vi "calculation vi_MD.vi"() -> ()   [LabVIEW 2012]
uses:
  Custom Controls/display palette control.ctl
  Custom Controls/scan mode main settings tab.ctl
  Custom Controls/pixel resolution enum.ctl
  Custom Controls/speed mode type def.ctl
  <vilib>/Utility/miscctls.llb/LVMinMaxIncTypeDef.ctl
  <vilib>/Utility/miscctls.llb/LVOutOfRangeActionTypeDef.ctl
  Custom Controls/experiment type.ctl
  Custom Controls/advanced settings inner tab CTL.ctl
  Custom Controls/MAIN Image panel tab Control type def.ctl
  Custom Controls/Histogram tab.ctl
  GFG/GFGnumericGet.vi
  GFG/GFGfpRefGet.vi
  GFG/GFGbooleanGet.vi
  GFG/GFGDisplayRefsGet.vi
  GFG/GFGImageRefsGet.vi
  GFG/GFG library.lvlib
panel:
  in  "String":string
  out "ready for flystart?":bool
  out "error out 2":errorcluster
  out "error out":errorcluster
  out "Source VI":string
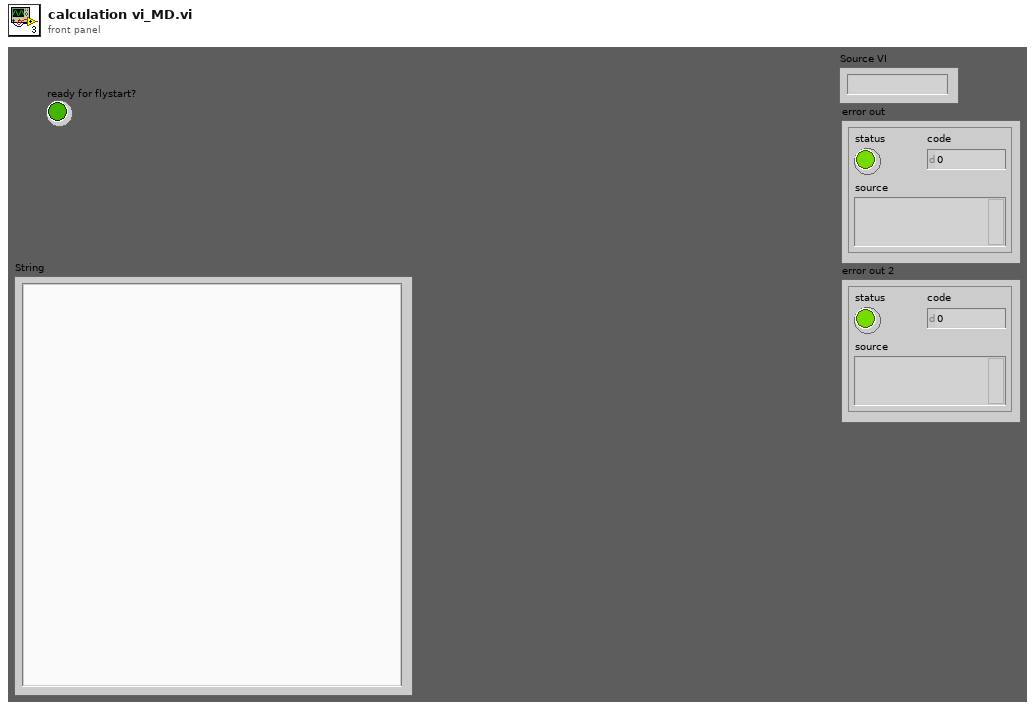
[diagram p1: front panel]
types:
  T1 = typedef "display palette control.ctl" = enum16{"standard", "high clipping red", "low clipping blue", "high and low clipping"}
  T2 = typedef "scan mode main settings tab.ctl" = enum32{"2D frame", "2D line scan", "general settings", "Z Stack", "piezo"}
  T3 = typedef "pixel resolution enum.ctl" = enum16{"   128 x 128", "   256 x 128", "   256 x 256", "   512 x  64", "   512 x 128", "   512 x 256", "   512 x 512", "  1024 x 512", "  1024 x 1024", "   arbitrary"}
  T4 = enum8{"Enabled", "Disabled", "Disabled and Grayed Out"}
  T5 = typedef "LVOutOfRangeActionTypeDef.ctl" = cluster{"Out of Range Action Minimum":u8, "Out of Range Action Maximum":u8, "Out of Range Action Increment":u8}
  T6 = typedef "LVMinMaxIncTypeDef.ctl" = cluster{"Minimum":dbl, "Maximum":dbl, "Increment":dbl}
  T7 = typedef "experiment type.ctl" = string
  T8 = enum32{"Page Enabled", "Page Disabled", "Page Disabled & Grayed"}
  T9 = typedef "advanced settings inner tab CTL.ctl" = enum32{"arb. frames", "AO", "AI", "channels", "trigger", "Zstack data"}
  T10 = typedef "MAIN Image panel tab Control type def.ctl" = enum32{"Channel 1", "Channel 2", "Channel 3", "Channel 4", "all channels", "RGB overlay", "ROI", "arbitrary line scan"}
  T11 = typedef "Histogram tab.ctl" = enum32{"hist Ch 1", "hist Ch 4", "hist Ch 3", "hist Ch 2"}
  T12 = cluster{"WaveformChartRef":refnum<vi>, "DigitalRef":refnum<vi>, "ArrayRef":refnum<vi>, "TabControlRef":refnum<vi>, "EnumRef":refnum<vi>, "RingRef":refnum<vi>, "BooleanRef":refnum<vi>, "KnobRef":refnum<vi>, "SlideRef":refnum<vi>, "PathRef":refnum<vi>, "StringRef":refnum<vi>, "ComboBox":refnum<vi>, "WaveformGraphRef":refnum<vi>}
  T13 = cluster{"Channel 1 small":refnum<vi>, "Channel 2 small":refnum<vi>, "Channel 3 small":refnum<vi>, "Channel 4 small":refnum<vi>, "Channel 1 large":refnum<vi>, "Channel 2 large":refnum<vi>, "Channel 3 large":refnum<vi>, "Channel 4 large":refnum<vi>, "RGB overlay":refnum<vi>, "ROI Image display":refnum<vi>, "arb line scan display":refnum<vi>, "Channel 5 large":refnum<vi>}
  T14 = typedef "IMAQ Image.ctl" = refnum<image>
  T15 = cluster{"Channel 1 small":T14, "Channel 2 small":T14, "Channel 3 small":T14, "Channel 4 small":T14, "Channel 1 large":T14, "Channel 2 large":T14, "Channel 3 large":T14, "Channel 4 large":T14, "RGB overlay":T14, "ROI Image display":T14, "arb line scan display":T14, "Channel 5 large":T14}
  T16 = typedef "speed mode type def.ctl" = u16
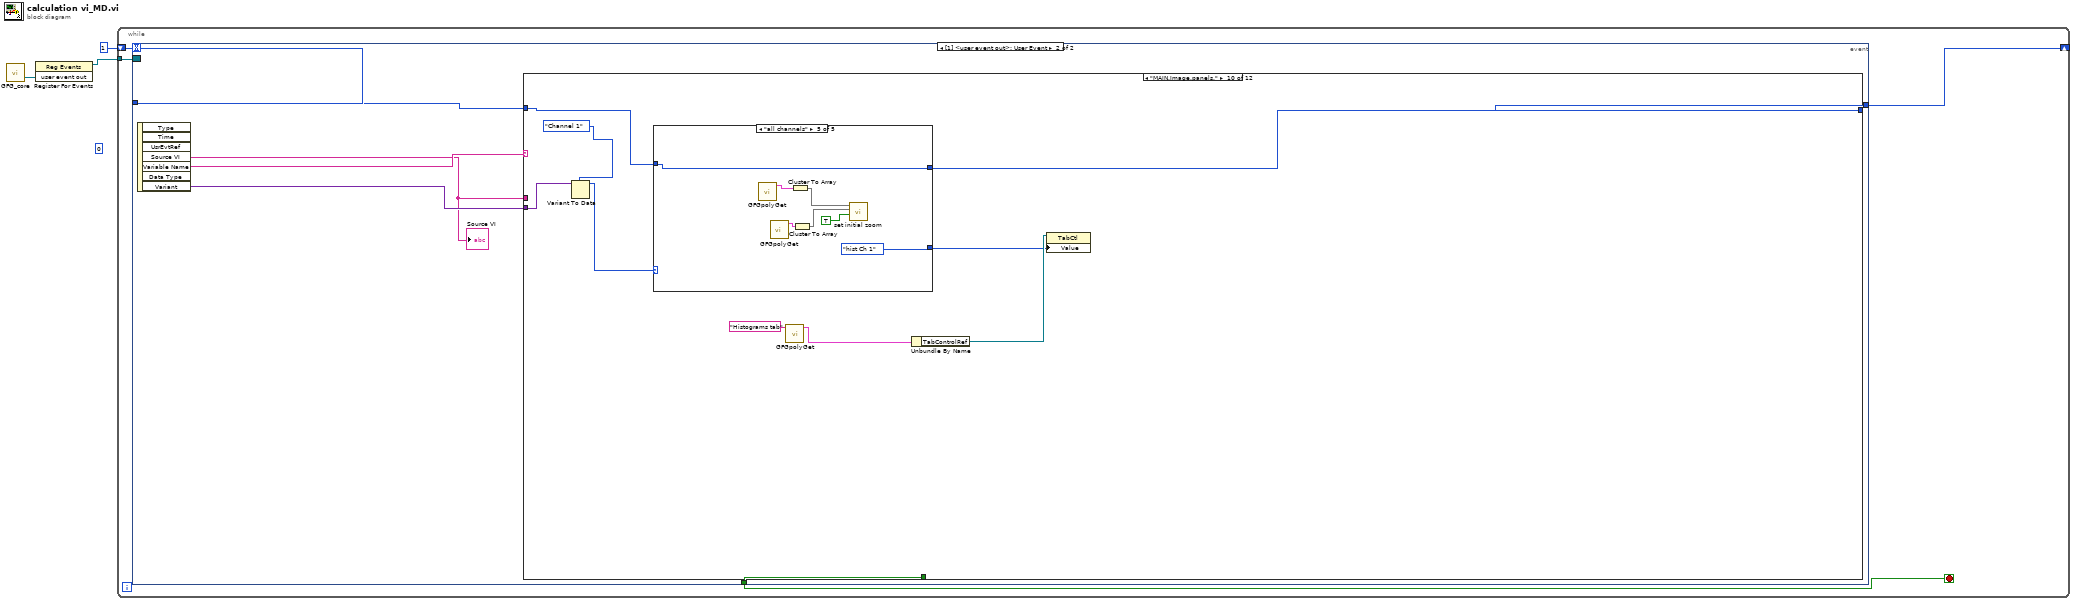
[diagram p0: block diagram]
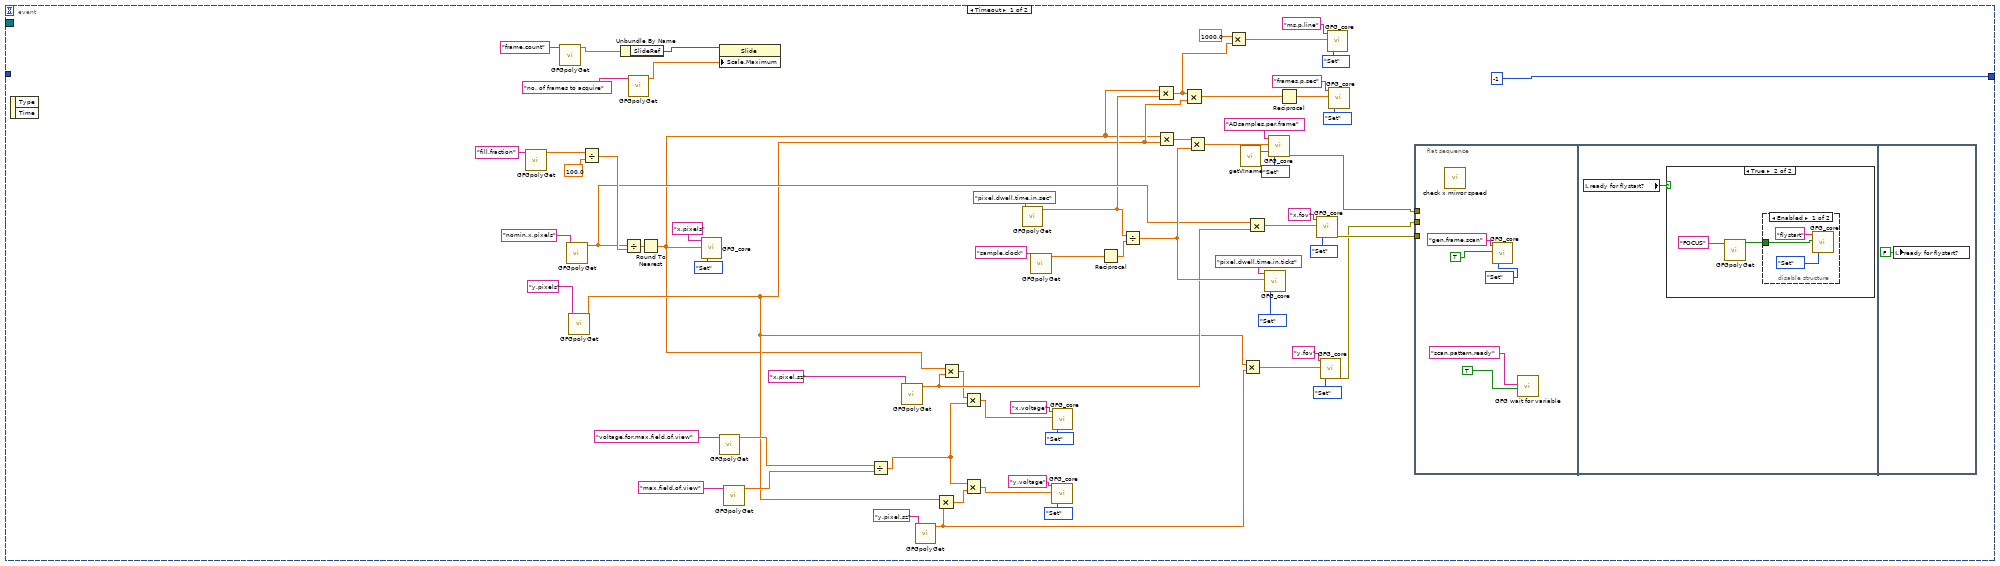
[diagram p2: hidden frame]
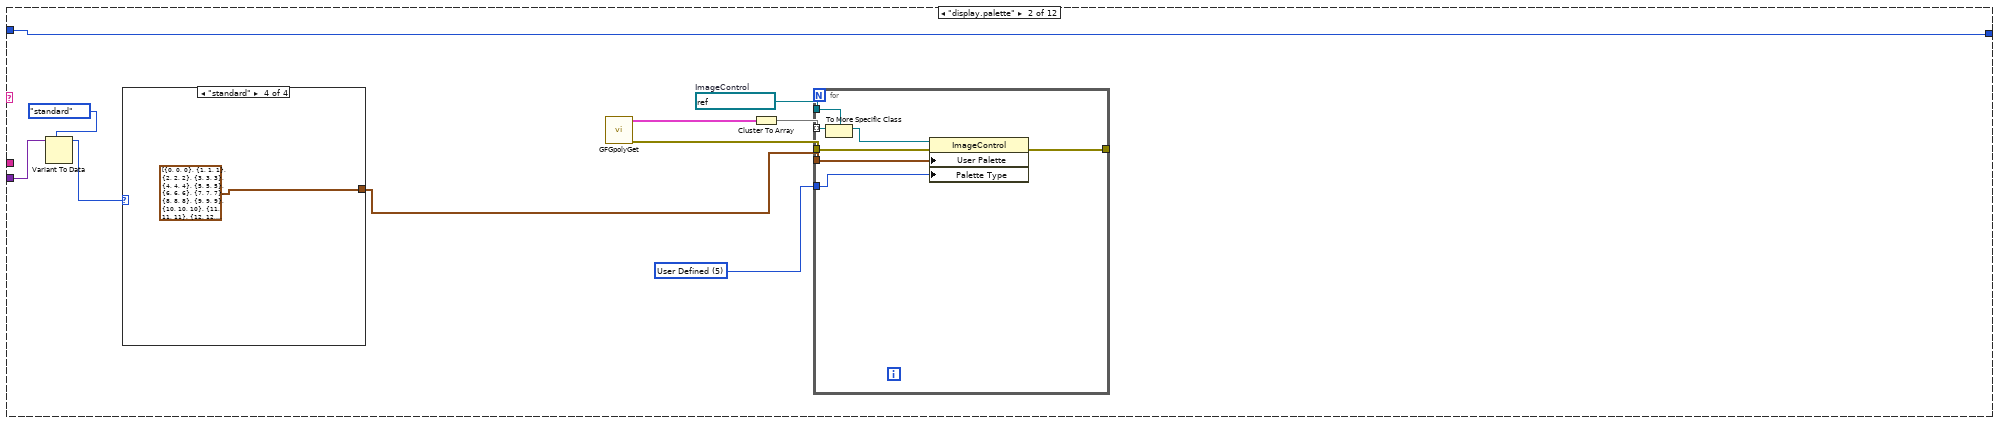
[diagram p6: hidden frame]
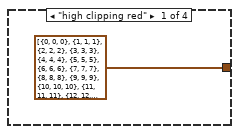
[diagram p7: hidden frame]
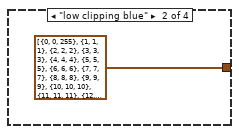
[diagram p8: hidden frame]
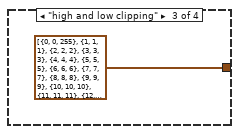
[diagram p9: hidden frame]
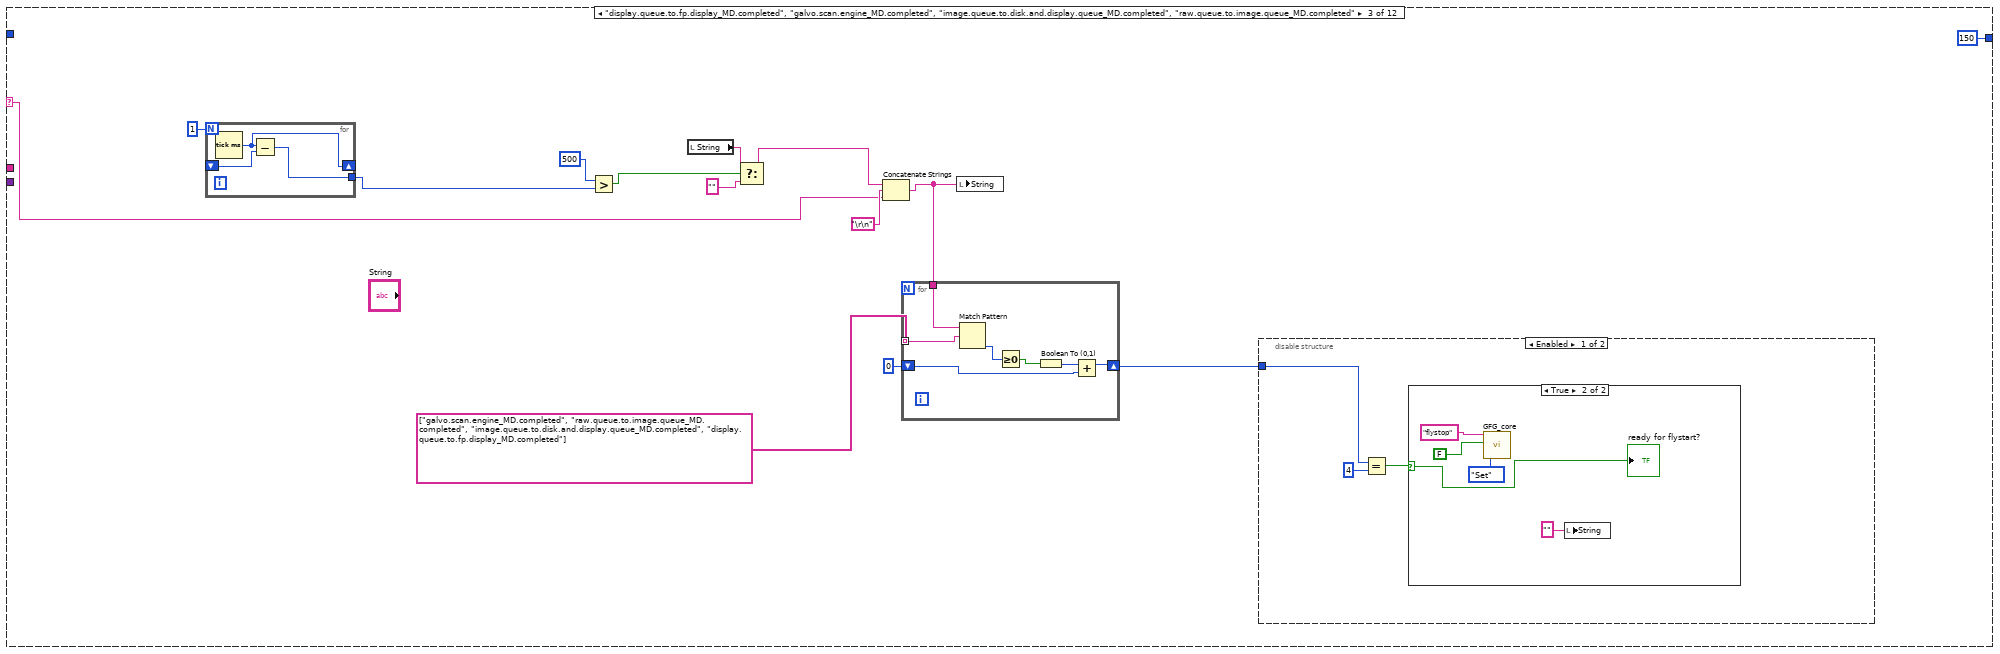
[diagram p10: hidden frame]
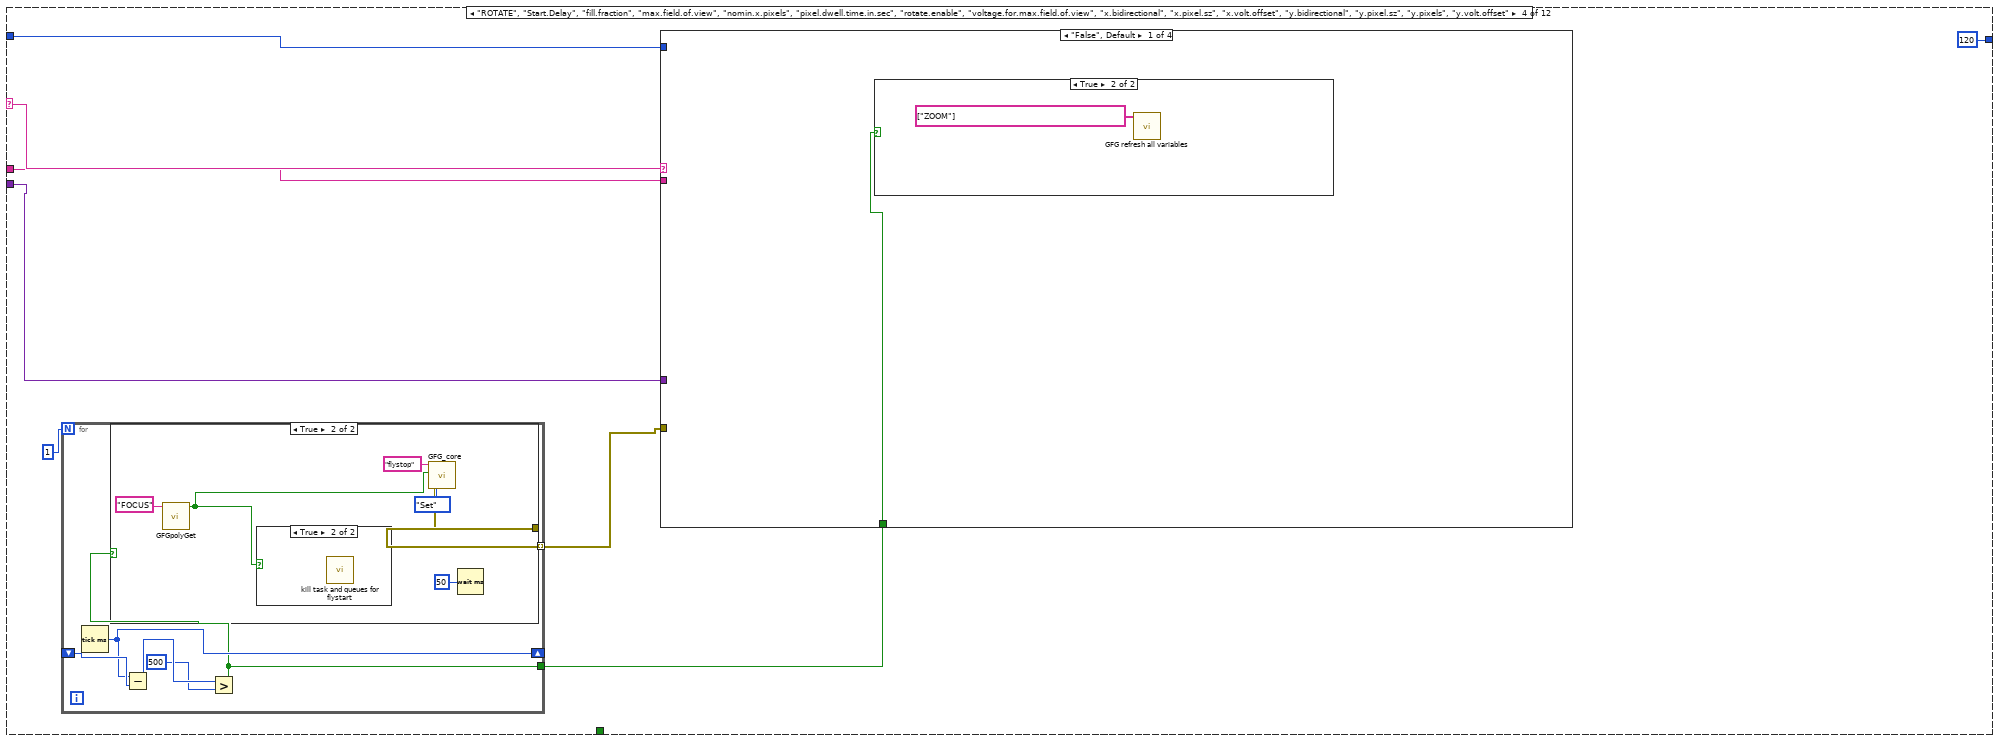
[diagram p13: hidden frame]
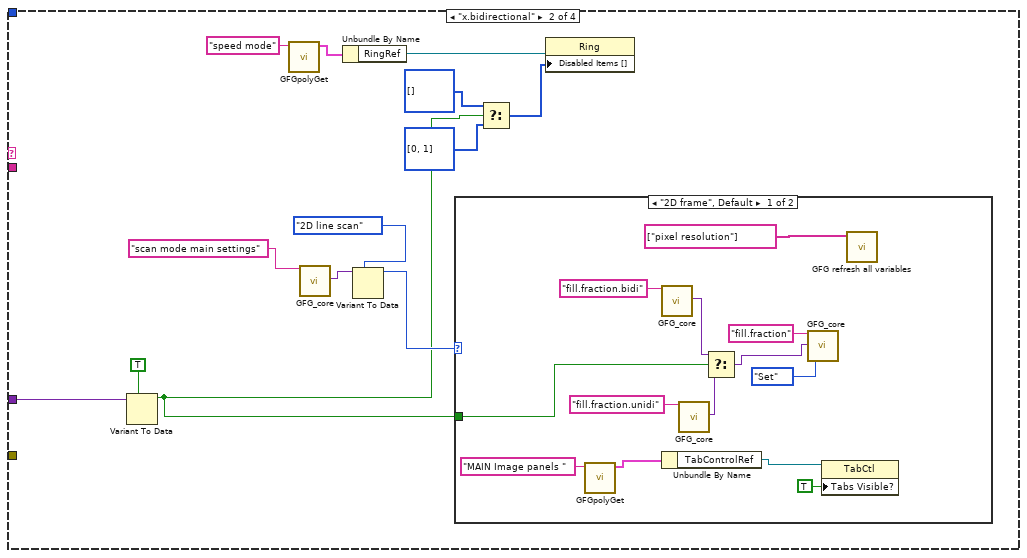
[diagram p17: hidden frame]
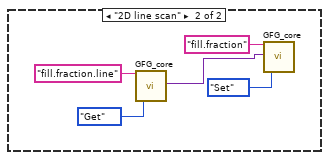
[diagram p18: hidden frame]
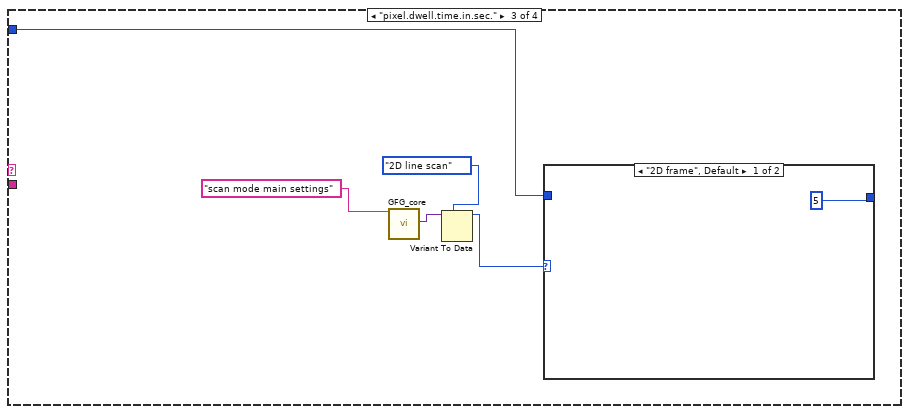
[diagram p19: hidden frame]
diagram:
  (unwired) 0
  n1 = call "GFG_core.vi"() -> ("user event out"=w3:refnum<user-event>)  [unwired: 13 in, 6 out]
  n2 = register-events(w3) -> (reference out=w2:refnum<event-registration>)  [unwired: 2 in, 1 out]
  n3 = while {
    tunnel: w2 -> [w7]
    shift-right: [w5] -> _
    shift-left: 1 -> [w4]
    stop <- w6 stop-if-true
    n4 = event shown="[1] <user event out>: User Event" {
      selector: w7 -> [_ _]
      dyn-events: _ -> [_ _]
      timeout: w4 -> [_ _]
      tunnel: [_ w90] -> w6
      tunnel: [-1 w88] -> w5
      tunnel: w4 -> [_ w87]
      event Timeout {
        n5 = event-data() -> ()  [unwired: 1 in, 2 out]
        n6 = call-poly "GFGpolyGet.vi"("Variable Name in"="fill.fraction") -> ("Numeric"=w53:dbl)  [unwired: 9 in, 1 out]
        n7 = call-poly "GFGpolyGet.vi"("Variable Name in"="frame.count") -> ("output cluster"=w14:T12)  [unwired: 9 in, 1 out]
        n8 = call-poly "GFGpolyGet.vi"("Variable Name in"="nomin.x.pixels") -> ("Numeric"=w29:dbl)  [unwired: 9 in, 1 out]
        n9 = call-poly "GFGpolyGet.vi"("Variable Name in"="y.pixels") -> ("Numeric"=w17:dbl)  [unwired: 9 in, 1 out]
        n10 = Divide(x=w53, y=100.0) -> (x/y=w49:dbl)
        n11 = Unbundle By Name(w14) -> ("SlideRef"=w13:refnum<vi>)
        n12 = Divide(x=w29, y=w49) -> (x/y=w30:dbl)
        n13 = call-poly "GFGpolyGet.vi"("Variable Name in"="no. of frames to acquire") -> ("Numeric"=w11:dbl)  [unwired: 9 in, 1 out]
        n14 = Round To Nearest(number=w30) -> (nearest integer value=w16:dbl)
        n15 = call "GFG_core.vi"("Variable Name in"="x.pixels", "Variant in"=w16, "Action"=enum16{"Init", "Set", "Get"}."Set") -> ()  [unwired: 10 in, 7 out]
        n16 = call-poly "GFGpolyGet.vi"("Variable Name in"="voltage.for.max.field.of.view") -> ("Numeric"=w44:dbl)  [unwired: 9 in, 1 out]
        n17 = property class="Slide"(reference=w13, "Scale.Maximum"=w11) -> ()  [unwired: 1 in, 2 out]
        n18 = call-poly "GFGpolyGet.vi"("Variable Name in"="max.field.of.view") -> ("Numeric"=w45:dbl)  [unwired: 9 in, 1 out]
        n19 = Divide(x=w44, y=w45) -> (x/y=w43:dbl)
        n20 = call-poly "GFGpolyGet.vi"("Variable Name in"="x.pixel.sz") -> ("Numeric"=w35:dbl)  [unwired: 9 in, 1 out]
        n21 = call-poly "GFGpolyGet.vi"("Variable Name in"="y.pixel.sz") -> ("Numeric"=w33:dbl)  [unwired: 9 in, 1 out]
        n22 = Multiply(x=w17, y=w33) -> (x*y=w32:dbl)
        n23 = Multiply(x=w16, y=w35) -> (x*y=w34:dbl)
        n24 = Multiply(x=w34, y=w43) -> (x*y=w38:dbl)
        n25 = Multiply(x=w43, y=w32) -> (x*y=w37:dbl)
        n26 = call-poly "GFGpolyGet.vi"("Variable Name in"="pixel.dwell.time.in.sec") -> ("Numeric"=w21:dbl)  [unwired: 9 in, 1 out]
        n27 = call-poly "GFGpolyGet.vi"("Variable Name in"="sample.clock") -> ("Numeric"=w31:dbl)  [unwired: 9 in, 1 out]
        n28 = call "GFG_core.vi"("Variable Name in"="y.voltage", "Variant in"=w37, "Action"=enum16{"Init", "Set", "Get"}."Set") -> ()  [unwired: 10 in, 7 out]
        n29 = call "GFG_core.vi"("Variable Name in"="x.voltage", "Variant in"=w38, "Action"=enum16{"Init", "Set", "Get"}."Set") -> ()  [unwired: 10 in, 7 out]
        n30 = Reciprocal(x=w31) -> (1/x=w60:dbl)
        n31 = Divide(x=w21, y=w60) -> (x/y=w56:dbl)
        n32 = Multiply(x=w16, y=w21) -> (x*y=w20:dbl)
        n33 = Multiply(x=w16, y=w17) -> (x*y=w28:dbl)
        n34 = Multiply(x=w20, y=w17) -> (x*y=w23:dbl)
        n35 = Multiply(x=w28, y=w56) -> (x*y=w72:dbl)
        n36 = Multiply(x=1000.0, y=w20) -> (x*y=w18:dbl)
        n37 = call "getVIname.vi"() -> ("VI name"=w70:string)  [unwired: 19 in]
        n38 = Multiply(x=w17, y=w33) -> (x*y=w62:dbl)
        n39 = Multiply(x=w29, y=w35) -> (x*y=w65:dbl)
        n40 = call "GFG_core.vi"("Variable Name in"="pixel.dwell.time.in.ticks", "Variant in"=w56, "Action"=enum16{"Init", "Set", "Get"}."Set") -> ()  [unwired: 10 in, 7 out]
        n41 = call "GFG_core.vi"("Variable Name in"="ADsamples.per.frame", "Variant in"=w72, "Source VI"=w70, "Action"=enum16{"Init", "Set", "Get"}."Set") -> ("error out"=w10:errorcluster)  [unwired: 9 in, 6 out]
        n42 = Reciprocal(x=w23) -> (1/x=w22:dbl)
        n43 = call "GFG_core.vi"("Variable Name in"="x.fov", "Variant in"=w65, "Action"=enum16{"Init", "Set", "Get"}."Set") -> ("error out"=w9:errorcluster)  [unwired: 10 in, 6 out]
        n44 = call "GFG_core.vi"("Variable Name in"="y.fov", "Variant in"=w62, "Action"=enum16{"Init", "Set", "Get"}."Set") -> ("error out"=w8:errorcluster)  [unwired: 10 in, 6 out]
        n45 = call "GFG_core.vi"("Variable Name in"="ms.p.line", "Variant in"=w18, "Action"=enum16{"Init", "Set", "Get"}."Set") -> ()  [unwired: 10 in, 7 out]
        n46 = call "GFG_core.vi"("Variable Name in"="frames.p.sec", "Variant in"=w22, "Action"=enum16{"Init", "Set", "Get"}."Set") -> ()  [unwired: 10 in, 7 out]
        n47 = flat-sequence {
          tunnel: w10 -> [_]
          tunnel: w9 -> [_]
          tunnel: w8 -> [_]
          frame #0 {
            n48 = call "check x mirror speed.vi"() -> ()  [unwired: 11 in, 1 out]
            n49 = call "GFG_core.vi"("Variable Name in"="gen.frame.scan", "Variant in"=TRUE, "Action"=enum16{"Init", "Set", "Get"}."Set") -> ()  [unwired: 10 in, 7 out]
            n50 = call "GFG wait for variable.vi"("Variant"=TRUE, "Variable Name"="scan.pattern.ready" ("Variable Name in")) -> ()  [unwired: 10 in]
          }
          frame #1 {
            n51 = local read "ready for flystart?"() -> (w79:bool)
            n52 = case shown="True" w79 {
              frame False {
              }
              frame True {
                n53 = call-poly "GFGpolyGet.vi"("Variable Name in"="FOCUS") -> ("Boolean"=w80:bool)  [unwired: 10 in]
                n54 = disable-structure shown="Enabled" {
                  disable-tunnel: w80 -> [w82 _]
                  frame Enabled {
                    n55 = call "GFG_core.vi"("Variable Name in"="flystart", "Variant in"=w82, "Action"=enum16{"Init", "Set", "Get"}."Set") -> ()  [unwired: 10 in, 7 out]
                  }
                  frame Disabled {
                  }
                }
              }
            }
          }
          frame #2 {
            n56 = local write "ready for flystart?"(FALSE ("ready for flystart?")) -> ()
          }
        }
      }
      event User Event {
        n57 = event-data() -> ("Source VI"=w86:string, "Variable Name"=w91:string, "Variant"=w89:variant)  [unwired: 1 in, 4 out]
        "Source VI" <- w86
        n58 = case shown="\"MAIN.Image.panels.\"" w91 {
          selector: w91 -> [_ _ w115 w153 _ _ w249 _ _ _ _ _]
          tunnel: [_ _ _ _ _ _ _ _ _ _ _ TRUE] -> w90
          tunnel: w89 -> [_ w97 _ w152 w233 _ w251 _ w380 w422 w456 _]
          tunnel: [w92 w93 150 120 w231 w240 120 w366 w376 w419 w457 w458] -> w88
          tunnel: w87 -> [w92 w93 _ w151 w231 w240 _ w366 w377 w420 w457 w458]
          tunnel: w86 -> [_ _ _ w150 _ _ _ _ _ _ _ _]
          frame "False", Default {
          }
          frame "display.palette" {
            w98 = u32 5 items=["Grayscale", "Binary", "Gradient", "Rainbow", "Temperature", "User Defined"] ("Palette:Palette Type")
            w100 = refnum<vi> refnum  # ImageControl
            n59 = Variant To Data(type=display_palette_control."standard" ("display palette"), Variant=w97) -> (data=w95:T1)  [unwired: 1 in, 1 out]
            n60 = case shown="\"standard\"" w95 {
              tunnel: [cluster{"Red":u8, "Green":u8, "Blue":u8}[] [{"Red"=0, "Green"=0, "Blue"=0}, {"Red"=1, "Green"=1, "Blue"=1}, {"Red"=2, "Green"=2, "Blue"=2}, {"Red"=3, "Green"=3, "Blue"=3}, {"Red"=4, "Green"=4, "Blue"=4}, {"Red"=5, "Green"=5, "Blue"=5}, {"Red"=6, "Green"=6, "Blue"=6}, {"Red"=7, "Green"=7, "Blue"=7}, {"Red"=8, "Green"=8, "Blue"=8}, {"Red"=9, "Green"=9, "Blue"=9}, {"Red"=10, "Green"=10, "Blue"=10}, {"Red"=11, "Green"=11, "Blue"=11}, {"Red"=12, "Green"=12, "Blue"=12}, {"Red"=13, "Green"=13, "Blue"=13}, {"Red"=14, "Green"=14, "Blue"=14}, {"Red"=15, "Green"=15, "Blue"=15}, {"Red"=16, "Green"=16, "Blue"=16}, {"Red"=17, "Green"=17, "Blue"=17}, {"Red"=18, "Green"=18, "Blue"=18}, {"Red"=19, "Green"=19, "Blue"=19}, {"Red"=20, "Green"=20, "Blue"=20}, {"Red"=21, "Green"=21, "Blue"=21}, {"Red"=22, "Green"=22, "Blue"=22}, {"Red"=23, "Green"=23, "Blue"=23}, {"Red"=24, "Green"=24, "Blue"=24}, {"Red"=25, "Green"=25, "Blue"=25}, {"Red"=26, "Green"=26, "Blue"=26}, {"Red"=27, "Green"=27, "Blue"=27}, {"Red"=28, "Green"=28, "Blue"=28}, {"Red"=29, "Green"=29, "Blue"=29}, {"Red"=30, "Green"=30, "Blue"=30}, {"Red"=31, "Green"=31, "Blue"=31}, {"Red"=32, "Green"=32, "Blue"=32}, {"Red"=33, "Green"=33, "Blue"=33}, {"Red"=34, "Green"=34, "Blue"=34}, {"Red"=35, "Green"=35, "Blue"=35}, {"Red"=36, "Green"=36, "Blue"=36}, {"Red"=37, "Green"=37, "Blue"=37}, {"Red"=38, "Green"=38, "Blue"=38}, {"Red"=39, "Green"=39, "Blue"=39}, {"Red"=40, "Green"=40, "Blue"=40}, {"Red"=41, "Green"=41, "Blue"=41}, {"Red"=42, "Green"=42, "Blue"=42}, {"Red"=43, "Green"=43, "Blue"=43}, {"Red"=44, "Green"=44, "Blue"=44}, {"Red"=45, "Green"=45, "Blue"=45}, {"Red"=46, "Green"=46, "Blue"=46}, {"Red"=47, "Green"=47, "Blue"=47}, {"Red"=48, "Green"=48, "Blue"=48}, {"Red"=49, "Green"=49, "Blue"=49}, {"Red"=50, "Green"=50, "Blue"=50}, {"Red"=51, "Green"=51, "Blue"=51}, {"Red"=52, "Green"=52, "Blue"=52}, {"Red"=53, "Green"=53, "Blue"=53}, {"Red"=54, "Green"=54, "Blue"=54}, {"Red"=55, "Green"=55, "Blue"=55}, {"Red"=56, "Green"=56, "Blue"=56}, {"Red"=57, "Green"=57, "Blue"=57}, {"Red"=58, "Green"=58, "Blue"=58}, {"Red"=59, "Green"=59, "Blue"=59}, {"Red"=60, "Green"=60, "Blue"=60}, {"Red"=61, "Green"=61, "Blue"=61}, {"Red"=62, "Green"=62, "Blue"=62}, {"Red"=63, "Green"=63, "Blue"=63}, {"Red"=64, "Green"=64, "Blue"=64}, {"Red"=65, "Green"=65, "Blue"=65}, {"Red"=66, "Green"=66, "Blue"=66}, {"Red"=67, "Green"=67, "Blue"=67}, {"Red"=68, "Green"=68, "Blue"=68}, {"Red"=69, "Green"=69, "Blue"=69}, {"Red"=70, "Green"=70, "Blue"=70}, {"Red"=71, "Green"=71, "Blue"=71}, {"Red"=72, "Green"=72, "Blue"=72}, {"Red"=73, "Green"=73, "Blue"=73}, {"Red"=74, "Green"=74, "Blue"=74}, {"Red"=75, "Green"=75, "Blue"=75}, {"Red"=76, "Green"=76, "Blue"=76}, {"Red"=77, "Green"=77, "Blue"=77}, {"Red"=78, "Green"=78, "Blue"=78}, {"Red"=79, "Green"=79, "Blue"=79}, {"Red"=80, "Green"=80, "Blue"=80}, {"Red"=81, "Green"=81, "Blue"=81}, {"Red"=82, "Green"=82, "Blue"=82}, {"Red"=83, "Green"=83, "Blue"=83}, {"Red"=84, "Green"=84, "Blue"=84}, {"Red"=85, "Green"=85, "Blue"=85}, {"Red"=86, "Green"=86, "Blue"=86}, {"Red"=87, "Green"=87, "Blue"=87}, {"Red"=88, "Green"=88, "Blue"=88}, {"Red"=89, "Green"=89, "Blue"=89}, {"Red"=90, "Green"=90, "Blue"=90}, {"Red"=91, "Green"=91, "Blue"=91}, {"Red"=92, "Green"=92, "Blue"=92}, {"Red"=93, "Green"=93, "Blue"=93}, {"Red"=94, "Green"=94, "Blue"=94}, {"Red"=95, "Green"=95, "Blue"=95}, {"Red"=96, "Green"=96, "Blue"=96}, {"Red"=97, "Green"=97, "Blue"=97}, {"Red"=98, "Green"=98, "Blue"=98}, {"Red"=99, "Green"=99, "Blue"=99}, {"Red"=100, "Green"=100, "Blue"=100}, {"Red"=101, "Green"=101, "Blue"=101}, {"Red"=102, "Green"=102, "Blue"=102}, {"Red"=103, "Green"=103, "Blue"=103}, {"Red"=104, "Green"=104, "Blue"=104}, {"Red"=105, "Green"=105, "Blue"=105}, {"Red"=106, "Green"=106, "Blue"=106}, {"Red"=107, "Green"=107, "Blue"=107}, {"Red"=108, "Green"=108, "Blue"=108}, {"Red"=109, "Green"=109, "Blue"=109}, {"Red"=110, "Green"=110, "Blue"=110}, {"Red"=111, "Green"=111, "Blue"=111}, {"Red"=112, "Green"=112, "Blue"=112}, {"Red"=113, "Green"=113, "Blue"=113}, {"Red"=114, "Green"=114, "Blue"=114}, {"Red"=115, "Green"=115, "Blue"=115}, {"Red"=116, "Green"=116, "Blue"=116}, {"Red"=117, "Green"=117, "Blue"=117}, {"Red"=118, "Green"=118, "Blue"=118}, {"Red"=119, "Green"=119, "Blue"=119}, {"Red"=120, "Green"=120, "Blue"=120}, {"Red"=121, "Green"=121, "Blue"=121}, {"Red"=122, "Green"=122, "Blue"=122}, {"Red"=123, "Green"=123, "Blue"=123}, {"Red"=124, "Green"=124, "Blue"=124}, {"Red"=125, "Green"=125, "Blue"=125}, {"Red"=126, "Green"=126, "Blue"=126}, {"Red"=127, "Green"=127, "Blue"=127}, {"Red"=128, "Green"=128, "Blue"=128}, {"Red"=129, "Green"=129, "Blue"=129}, {"Red"=130, "Green"=130, "Blue"=130}, {"Red"=131, "Green"=131, "Blue"=131}, {"Red"=132, "Green"=132, "Blue"=132}, {"Red"=133, "Green"=133, "Blue"=133}, {"Red"=134, "Green"=134, "Blue"=134}, {"Red"=135, "Green"=135, "Blue"=135}, {"Red"=136, "Green"=136, "Blue"=136}, {"Red"=137, "Green"=137, "Blue"=137}, {"Red"=138, "Green"=138, "Blue"=138}, {"Red"=139, "Green"=139, "Blue"=139}, {"Red"=140, "Green"=140, "Blue"=140}, {"Red"=141, "Green"=141, "Blue"=141}, {"Red"=142, "Green"=142, "Blue"=142}, {"Red"=143, "Green"=143, "Blue"=143}, {"Red"=144, "Green"=144, "Blue"=144}, {"Red"=145, "Green"=145, "Blue"=145}, {"Red"=146, "Green"=146, "Blue"=146}, {"Red"=147, "Green"=147, "Blue"=147}, {"Red"=148, "Green"=148, "Blue"=148}, {"Red"=149, "Green"=149, "Blue"=149}, {"Red"=150, "Green"=150, "Blue"=150}, {"Red"=151, "Green"=151, "Blue"=151}, {"Red"=152, "Green"=152, "Blue"=152}, {"Red"=153, "Green"=153, "Blue"=153}, {"Red"=154, "Green"=154, "Blue"=154}, {"Red"=155, "Green"=155, "Blue"=155}, {"Red"=156, "Green"=156, "Blue"=156}, {"Red"=157, "Green"=157, "Blue"=157}, {"Red"=158, "Green"=158, "Blue"=158}, {"Red"=159, "Green"=159, "Blue"=159}, {"Red"=160, "Green"=160, "Blue"=160}, {"Red"=161, "Green"=161, "Blue"=161}, {"Red"=162, "Green"=162, "Blue"=162}, {"Red"=163, "Green"=163, "Blue"=163}, {"Red"=164, "Green"=164, "Blue"=164}, {"Red"=165, "Green"=165, "Blue"=165}, {"Red"=166, "Green"=166, "Blue"=166}, {"Red"=167, "Green"=167, "Blue"=167}, {"Red"=168, "Green"=168, "Blue"=168}, {"Red"=169, "Green"=169, "Blue"=169}, {"Red"=170, "Green"=170, "Blue"=170}, {"Red"=171, "Green"=171, "Blue"=171}, {"Red"=172, "Green"=172, "Blue"=172}, {"Red"=173, "Green"=173, "Blue"=173}, {"Red"=174, "Green"=174, "Blue"=174}, {"Red"=175, "Green"=175, "Blue"=175}, {"Red"=176, "Green"=176, "Blue"=176}, {"Red"=177, "Green"=177, "Blue"=177}, {"Red"=178, "Green"=178, "Blue"=178}, {"Red"=179, "Green"=179, "Blue"=179}, {"Red"=180, "Green"=180, "Blue"=180}, {"Red"=181, "Green"=181, "Blue"=181}, {"Red"=182, "Green"=182, "Blue"=182}, {"Red"=183, "Green"=183, "Blue"=183}, {"Red"=184, "Green"=184, "Blue"=184}, {"Red"=185, "Green"=185, "Blue"=185}, {"Red"=186, "Green"=186, "Blue"=186}, {"Red"=187, "Green"=187, "Blue"=187}, {"Red"=188, "Green"=188, "Blue"=188}, {"Red"=189, "Green"=189, "Blue"=189}, {"Red"=190, "Green"=190, "Blue"=190}, {"Red"=191, "Green"=191, "Blue"=191}, {"Red"=192, "Green"=192, "Blue"=192}, {"Red"=193, "Green"=193, "Blue"=193}, {"Red"=194, "Green"=194, "Blue"=194}, {"Red"=195, "Green"=195, "Blue"=195}, {"Red"=196, "Green"=196, "Blue"=196}, {"Red"=197, "Green"=197, "Blue"=197}, {"Red"=198, "Green"=198, "Blue"=198}, {"Red"=199, "Green"=199, "Blue"=199}, {"Red"=200, "Green"=200, "Blue"=200}, {"Red"=201, "Green"=201, "Blue"=201}, {"Red"=202, "Green"=202, "Blue"=202}, {"Red"=203, "Green"=203, "Blue"=203}, {"Red"=204, "Green"=204, "Blue"=204}, {"Red"=205, "Green"=205, "Blue"=205}, {"Red"=206, "Green"=206, "Blue"=206}, {"Red"=207, "Green"=207, "Blue"=207}, {"Red"=208, "Green"=208, "Blue"=208}, {"Red"=209, "Green"=209, "Blue"=209}, {"Red"=210, "Green"=210, "Blue"=210}, {"Red"=211, "Green"=211, "Blue"=211}, {"Red"=212, "Green"=212, "Blue"=212}, {"Red"=213, "Green"=213, "Blue"=213}, {"Red"=214, "Green"=214, "Blue"=214}, {"Red"=215, "Green"=215, "Blue"=215}, {"Red"=216, "Green"=216, "Blue"=216}, {"Red"=217, "Green"=217, "Blue"=217}, {"Red"=218, "Green"=218, "Blue"=218}, {"Red"=219, "Green"=219, "Blue"=219}, {"Red"=220, "Green"=220, "Blue"=220}, {"Red"=221, "Green"=221, "Blue"=221}, {"Red"=222, "Green"=222, "Blue"=222}, {"Red"=223, "Green"=223, "Blue"=223}, {"Red"=224, "Green"=224, "Blue"=224}, {"Red"=225, "Green"=225, "Blue"=225}, {"Red"=226, "Green"=226, "Blue"=226}, {"Red"=227, "Green"=227, "Blue"=227}, {"Red"=228, "Green"=228, "Blue"=228}, {"Red"=229, "Green"=229, "Blue"=229}, {"Red"=230, "Green"=230, "Blue"=230}, {"Red"=231, "Green"=231, "Blue"=231}, {"Red"=232, "Green"=232, "Blue"=232}, {"Red"=233, "Green"=233, "Blue"=233}, {"Red"=234, "Green"=234, "Blue"=234}, {"Red"=235, "Green"=235, "Blue"=235}, {"Red"=236, "Green"=236, "Blue"=236}, {"Red"=237, "Green"=237, "Blue"=237}, {"Red"=238, "Green"=238, "Blue"=238}, {"Red"=239, "Green"=239, "Blue"=239}, {"Red"=240, "Green"=240, "Blue"=240}, {"Red"=241, "Green"=241, "Blue"=241}, {"Red"=242, "Green"=242, "Blue"=242}, {"Red"=243, "Green"=243, "Blue"=243}, {"Red"=244, "Green"=244, "Blue"=244}, {"Red"=245, "Green"=245, "Blue"=245}, {"Red"=246, "Green"=246, "Blue"=246}, {"Red"=247, "Green"=247, "Blue"=247}, {"Red"=248, "Green"=248, "Blue"=248}, {"Red"=249, "Green"=249, "Blue"=249}, {"Red"=250, "Green"=250, "Blue"=250}, {"Red"=251, "Green"=251, "Blue"=251}, {"Red"=252, "Green"=252, "Blue"=252}, {"Red"=253, "Green"=253, "Blue"=253}, {"Red"=254, "Green"=254, "Blue"=254}, {"Red"=255, "Green"=0, "Blue"=0}] ("Color Palette") cluster{"Red":u8, "Green":u8, "Blue":u8}[] [{"Red"=0, "Green"=0, "Blue"=255}, {"Red"=1, "Green"=1, "Blue"=1}, {"Red"=2, "Green"=2, "Blue"=2}, {"Red"=3, "Green"=3, "Blue"=3}, {"Red"=4, "Green"=4, "Blue"=4}, {"Red"=5, "Green"=5, "Blue"=5}, {"Red"=6, "Green"=6, "Blue"=6}, {"Red"=7, "Green"=7, "Blue"=7}, {"Red"=8, "Green"=8, "Blue"=8}, {"Red"=9, "Green"=9, "Blue"=9}, {"Red"=10, "Green"=10, "Blue"=10}, {"Red"=11, "Green"=11, "Blue"=11}, {"Red"=12, "Green"=12, "Blue"=12}, {"Red"=13, "Green"=13, "Blue"=13}, {"Red"=14, "Green"=14, "Blue"=14}, {"Red"=15, "Green"=15, "Blue"=15}, {"Red"=16, "Green"=16, "Blue"=16}, {"Red"=17, "Green"=17, "Blue"=17}, {"Red"=18, "Green"=18, "Blue"=18}, {"Red"=19, "Green"=19, "Blue"=19}, {"Red"=20, "Green"=20, "Blue"=20}, {"Red"=21, "Green"=21, "Blue"=21}, {"Red"=22, "Green"=22, "Blue"=22}, {"Red"=23, "Green"=23, "Blue"=23}, {"Red"=24, "Green"=24, "Blue"=24}, {"Red"=25, "Green"=25, "Blue"=25}, {"Red"=26, "Green"=26, "Blue"=26}, {"Red"=27, "Green"=27, "Blue"=27}, {"Red"=28, "Green"=28, "Blue"=28}, {"Red"=29, "Green"=29, "Blue"=29}, {"Red"=30, "Green"=30, "Blue"=30}, {"Red"=31, "Green"=31, "Blue"=31}, {"Red"=32, "Green"=32, "Blue"=32}, {"Red"=33, "Green"=33, "Blue"=33}, {"Red"=34, "Green"=34, "Blue"=34}, {"Red"=35, "Green"=35, "Blue"=35}, {"Red"=36, "Green"=36, "Blue"=36}, {"Red"=37, "Green"=37, "Blue"=37}, {"Red"=38, "Green"=38, "Blue"=38}, {"Red"=39, "Green"=39, "Blue"=39}, {"Red"=40, "Green"=40, "Blue"=40}, {"Red"=41, "Green"=41, "Blue"=41}, {"Red"=42, "Green"=42, "Blue"=42}, {"Red"=43, "Green"=43, "Blue"=43}, {"Red"=44, "Green"=44, "Blue"=44}, {"Red"=45, "Green"=45, "Blue"=45}, {"Red"=46, "Green"=46, "Blue"=46}, {"Red"=47, "Green"=47, "Blue"=47}, {"Red"=48, "Green"=48, "Blue"=48}, {"Red"=49, "Green"=49, "Blue"=49}, {"Red"=50, "Green"=50, "Blue"=50}, {"Red"=51, "Green"=51, "Blue"=51}, {"Red"=52, "Green"=52, "Blue"=52}, {"Red"=53, "Green"=53, "Blue"=53}, {"Red"=54, "Green"=54, "Blue"=54}, {"Red"=55, "Green"=55, "Blue"=55}, {"Red"=56, "Green"=56, "Blue"=56}, {"Red"=57, "Green"=57, "Blue"=57}, {"Red"=58, "Green"=58, "Blue"=58}, {"Red"=59, "Green"=59, "Blue"=59}, {"Red"=60, "Green"=60, "Blue"=60}, {"Red"=61, "Green"=61, "Blue"=61}, {"Red"=62, "Green"=62, "Blue"=62}, {"Red"=63, "Green"=63, "Blue"=63}, {"Red"=64, "Green"=64, "Blue"=64}, {"Red"=65, "Green"=65, "Blue"=65}, {"Red"=66, "Green"=66, "Blue"=66}, {"Red"=67, "Green"=67, "Blue"=67}, {"Red"=68, "Green"=68, "Blue"=68}, {"Red"=69, "Green"=69, "Blue"=69}, {"Red"=70, "Green"=70, "Blue"=70}, {"Red"=71, "Green"=71, "Blue"=71}, {"Red"=72, "Green"=72, "Blue"=72}, {"Red"=73, "Green"=73, "Blue"=73}, {"Red"=74, "Green"=74, "Blue"=74}, {"Red"=75, "Green"=75, "Blue"=75}, {"Red"=76, "Green"=76, "Blue"=76}, {"Red"=77, "Green"=77, "Blue"=77}, {"Red"=78, "Green"=78, "Blue"=78}, {"Red"=79, "Green"=79, "Blue"=79}, {"Red"=80, "Green"=80, "Blue"=80}, {"Red"=81, "Green"=81, "Blue"=81}, {"Red"=82, "Green"=82, "Blue"=82}, {"Red"=83, "Green"=83, "Blue"=83}, {"Red"=84, "Green"=84, "Blue"=84}, {"Red"=85, "Green"=85, "Blue"=85}, {"Red"=86, "Green"=86, "Blue"=86}, {"Red"=87, "Green"=87, "Blue"=87}, {"Red"=88, "Green"=88, "Blue"=88}, {"Red"=89, "Green"=89, "Blue"=89}, {"Red"=90, "Green"=90, "Blue"=90}, {"Red"=91, "Green"=91, "Blue"=91}, {"Red"=92, "Green"=92, "Blue"=92}, {"Red"=93, "Green"=93, "Blue"=93}, {"Red"=94, "Green"=94, "Blue"=94}, {"Red"=95, "Green"=95, "Blue"=95}, {"Red"=96, "Green"=96, "Blue"=96}, {"Red"=97, "Green"=97, "Blue"=97}, {"Red"=98, "Green"=98, "Blue"=98}, {"Red"=99, "Green"=99, "Blue"=99}, {"Red"=100, "Green"=100, "Blue"=100}, {"Red"=101, "Green"=101, "Blue"=101}, {"Red"=102, "Green"=102, "Blue"=102}, {"Red"=103, "Green"=103, "Blue"=103}, {"Red"=104, "Green"=104, "Blue"=104}, {"Red"=105, "Green"=105, "Blue"=105}, {"Red"=106, "Green"=106, "Blue"=106}, {"Red"=107, "Green"=107, "Blue"=107}, {"Red"=108, "Green"=108, "Blue"=108}, {"Red"=109, "Green"=109, "Blue"=109}, {"Red"=110, "Green"=110, "Blue"=110}, {"Red"=111, "Green"=111, "Blue"=111}, {"Red"=112, "Green"=112, "Blue"=112}, {"Red"=113, "Green"=113, "Blue"=113}, {"Red"=114, "Green"=114, "Blue"=114}, {"Red"=115, "Green"=115, "Blue"=115}, {"Red"=116, "Green"=116, "Blue"=116}, {"Red"=117, "Green"=117, "Blue"=117}, {"Red"=118, "Green"=118, "Blue"=118}, {"Red"=119, "Green"=119, "Blue"=119}, {"Red"=120, "Green"=120, "Blue"=120}, {"Red"=121, "Green"=121, "Blue"=121}, {"Red"=122, "Green"=122, "Blue"=122}, {"Red"=123, "Green"=123, "Blue"=123}, {"Red"=124, "Green"=124, "Blue"=124}, {"Red"=125, "Green"=125, "Blue"=125}, {"Red"=126, "Green"=126, "Blue"=126}, {"Red"=127, "Green"=127, "Blue"=127}, {"Red"=128, "Green"=128, "Blue"=128}, {"Red"=129, "Green"=129, "Blue"=129}, {"Red"=130, "Green"=130, "Blue"=130}, {"Red"=131, "Green"=131, "Blue"=131}, {"Red"=132, "Green"=132, "Blue"=132}, {"Red"=133, "Green"=133, "Blue"=133}, {"Red"=134, "Green"=134, "Blue"=134}, {"Red"=135, "Green"=135, "Blue"=135}, {"Red"=136, "Green"=136, "Blue"=136}, {"Red"=137, "Green"=137, "Blue"=137}, {"Red"=138, "Green"=138, "Blue"=138}, {"Red"=139, "Green"=139, "Blue"=139}, {"Red"=140, "Green"=140, "Blue"=140}, {"Red"=141, "Green"=141, "Blue"=141}, {"Red"=142, "Green"=142, "Blue"=142}, {"Red"=143, "Green"=143, "Blue"=143}, {"Red"=144, "Green"=144, "Blue"=144}, {"Red"=145, "Green"=145, "Blue"=145}, {"Red"=146, "Green"=146, "Blue"=146}, {"Red"=147, "Green"=147, "Blue"=147}, {"Red"=148, "Green"=148, "Blue"=148}, {"Red"=149, "Green"=149, "Blue"=149}, {"Red"=150, "Green"=150, "Blue"=150}, {"Red"=151, "Green"=151, "Blue"=151}, {"Red"=152, "Green"=152, "Blue"=152}, {"Red"=153, "Green"=153, "Blue"=153}, {"Red"=154, "Green"=154, "Blue"=154}, {"Red"=155, "Green"=155, "Blue"=155}, {"Red"=156, "Green"=156, "Blue"=156}, {"Red"=157, "Green"=157, "Blue"=157}, {"Red"=158, "Green"=158, "Blue"=158}, {"Red"=159, "Green"=159, "Blue"=159}, {"Red"=160, "Green"=160, "Blue"=160}, {"Red"=161, "Green"=161, "Blue"=161}, {"Red"=162, "Green"=162, "Blue"=162}, {"Red"=163, "Green"=163, "Blue"=163}, {"Red"=164, "Green"=164, "Blue"=164}, {"Red"=165, "Green"=165, "Blue"=165}, {"Red"=166, "Green"=166, "Blue"=166}, {"Red"=167, "Green"=167, "Blue"=167}, {"Red"=168, "Green"=168, "Blue"=168}, {"Red"=169, "Green"=169, "Blue"=169}, {"Red"=170, "Green"=170, "Blue"=170}, {"Red"=171, "Green"=171, "Blue"=171}, {"Red"=172, "Green"=172, "Blue"=172}, {"Red"=173, "Green"=173, "Blue"=173}, {"Red"=174, "Green"=174, "Blue"=174}, {"Red"=175, "Green"=175, "Blue"=175}, {"Red"=176, "Green"=176, "Blue"=176}, {"Red"=177, "Green"=177, "Blue"=177}, {"Red"=178, "Green"=178, "Blue"=178}, {"Red"=179, "Green"=179, "Blue"=179}, {"Red"=180, "Green"=180, "Blue"=180}, {"Red"=181, "Green"=181, "Blue"=181}, {"Red"=182, "Green"=182, "Blue"=182}, {"Red"=183, "Green"=183, "Blue"=183}, {"Red"=184, "Green"=184, "Blue"=184}, {"Red"=185, "Green"=185, "Blue"=185}, {"Red"=186, "Green"=186, "Blue"=186}, {"Red"=187, "Green"=187, "Blue"=187}, {"Red"=188, "Green"=188, "Blue"=188}, {"Red"=189, "Green"=189, "Blue"=189}, {"Red"=190, "Green"=190, "Blue"=190}, {"Red"=191, "Green"=191, "Blue"=191}, {"Red"=192, "Green"=192, "Blue"=192}, {"Red"=193, "Green"=193, "Blue"=193}, {"Red"=194, "Green"=194, "Blue"=194}, {"Red"=195, "Green"=195, "Blue"=195}, {"Red"=196, "Green"=196, "Blue"=196}, {"Red"=197, "Green"=197, "Blue"=197}, {"Red"=198, "Green"=198, "Blue"=198}, {"Red"=199, "Green"=199, "Blue"=199}, {"Red"=200, "Green"=200, "Blue"=200}, {"Red"=201, "Green"=201, "Blue"=201}, {"Red"=202, "Green"=202, "Blue"=202}, {"Red"=203, "Green"=203, "Blue"=203}, {"Red"=204, "Green"=204, "Blue"=204}, {"Red"=205, "Green"=205, "Blue"=205}, {"Red"=206, "Green"=206, "Blue"=206}, {"Red"=207, "Green"=207, "Blue"=207}, {"Red"=208, "Green"=208, "Blue"=208}, {"Red"=209, "Green"=209, "Blue"=209}, {"Red"=210, "Green"=210, "Blue"=210}, {"Red"=211, "Green"=211, "Blue"=211}, {"Red"=212, "Green"=212, "Blue"=212}, {"Red"=213, "Green"=213, "Blue"=213}, {"Red"=214, "Green"=214, "Blue"=214}, {"Red"=215, "Green"=215, "Blue"=215}, {"Red"=216, "Green"=216, "Blue"=216}, {"Red"=217, "Green"=217, "Blue"=217}, {"Red"=218, "Green"=218, "Blue"=218}, {"Red"=219, "Green"=219, "Blue"=219}, {"Red"=220, "Green"=220, "Blue"=220}, {"Red"=221, "Green"=221, "Blue"=221}, {"Red"=222, "Green"=222, "Blue"=222}, {"Red"=223, "Green"=223, "Blue"=223}, {"Red"=224, "Green"=224, "Blue"=224}, {"Red"=225, "Green"=225, "Blue"=225}, {"Red"=226, "Green"=226, "Blue"=226}, {"Red"=227, "Green"=227, "Blue"=227}, {"Red"=228, "Green"=228, "Blue"=228}, {"Red"=229, "Green"=229, "Blue"=229}, {"Red"=230, "Green"=230, "Blue"=230}, {"Red"=231, "Green"=231, "Blue"=231}, {"Red"=232, "Green"=232, "Blue"=232}, {"Red"=233, "Green"=233, "Blue"=233}, {"Red"=234, "Green"=234, "Blue"=234}, {"Red"=235, "Green"=235, "Blue"=235}, {"Red"=236, "Green"=236, "Blue"=236}, {"Red"=237, "Green"=237, "Blue"=237}, {"Red"=238, "Green"=238, "Blue"=238}, {"Red"=239, "Green"=239, "Blue"=239}, {"Red"=240, "Green"=240, "Blue"=240}, {"Red"=241, "Green"=241, "Blue"=241}, {"Red"=242, "Green"=242, "Blue"=242}, {"Red"=243, "Green"=243, "Blue"=243}, {"Red"=244, "Green"=244, "Blue"=244}, {"Red"=245, "Green"=245, "Blue"=245}, {"Red"=246, "Green"=246, "Blue"=246}, {"Red"=247, "Green"=247, "Blue"=247}, {"Red"=248, "Green"=248, "Blue"=248}, {"Red"=249, "Green"=249, "Blue"=249}, {"Red"=250, "Green"=250, "Blue"=250}, {"Red"=251, "Green"=251, "Blue"=251}, {"Red"=252, "Green"=252, "Blue"=252}, {"Red"=253, "Green"=253, "Blue"=253}, {"Red"=254, "Green"=254, "Blue"=254}, {"Red"=255, "Green"=255, "Blue"=255}] ("Color Palette") cluster{"Red":u8, "Green":u8, "Blue":u8}[] [{"Red"=0, "Green"=0, "Blue"=255}, {"Red"=1, "Green"=1, "Blue"=1}, {"Red"=2, "Green"=2, "Blue"=2}, {"Red"=3, "Green"=3, "Blue"=3}, {"Red"=4, "Green"=4, "Blue"=4}, {"Red"=5, "Green"=5, "Blue"=5}, {"Red"=6, "Green"=6, "Blue"=6}, {"Red"=7, "Green"=7, "Blue"=7}, {"Red"=8, "Green"=8, "Blue"=8}, {"Red"=9, "Green"=9, "Blue"=9}, {"Red"=10, "Green"=10, "Blue"=10}, {"Red"=11, "Green"=11, "Blue"=11}, {"Red"=12, "Green"=12, "Blue"=12}, {"Red"=13, "Green"=13, "Blue"=13}, {"Red"=14, "Green"=14, "Blue"=14}, {"Red"=15, "Green"=15, "Blue"=15}, {"Red"=16, "Green"=16, "Blue"=16}, {"Red"=17, "Green"=17, "Blue"=17}, {"Red"=18, "Green"=18, "Blue"=18}, {"Red"=19, "Green"=19, "Blue"=19}, {"Red"=20, "Green"=20, "Blue"=20}, {"Red"=21, "Green"=21, "Blue"=21}, {"Red"=22, "Green"=22, "Blue"=22}, {"Red"=23, "Green"=23, "Blue"=23}, {"Red"=24, "Green"=24, "Blue"=24}, {"Red"=25, "Green"=25, "Blue"=25}, {"Red"=26, "Green"=26, "Blue"=26}, {"Red"=27, "Green"=27, "Blue"=27}, {"Red"=28, "Green"=28, "Blue"=28}, {"Red"=29, "Green"=29, "Blue"=29}, {"Red"=30, "Green"=30, "Blue"=30}, {"Red"=31, "Green"=31, "Blue"=31}, {"Red"=32, "Green"=32, "Blue"=32}, {"Red"=33, "Green"=33, "Blue"=33}, {"Red"=34, "Green"=34, "Blue"=34}, {"Red"=35, "Green"=35, "Blue"=35}, {"Red"=36, "Green"=36, "Blue"=36}, {"Red"=37, "Green"=37, "Blue"=37}, {"Red"=38, "Green"=38, "Blue"=38}, {"Red"=39, "Green"=39, "Blue"=39}, {"Red"=40, "Green"=40, "Blue"=40}, {"Red"=41, "Green"=41, "Blue"=41}, {"Red"=42, "Green"=42, "Blue"=42}, {"Red"=43, "Green"=43, "Blue"=43}, {"Red"=44, "Green"=44, "Blue"=44}, {"Red"=45, "Green"=45, "Blue"=45}, {"Red"=46, "Green"=46, "Blue"=46}, {"Red"=47, "Green"=47, "Blue"=47}, {"Red"=48, "Green"=48, "Blue"=48}, {"Red"=49, "Green"=49, "Blue"=49}, {"Red"=50, "Green"=50, "Blue"=50}, {"Red"=51, "Green"=51, "Blue"=51}, {"Red"=52, "Green"=52, "Blue"=52}, {"Red"=53, "Green"=53, "Blue"=53}, {"Red"=54, "Green"=54, "Blue"=54}, {"Red"=55, "Green"=55, "Blue"=55}, {"Red"=56, "Green"=56, "Blue"=56}, {"Red"=57, "Green"=57, "Blue"=57}, {"Red"=58, "Green"=58, "Blue"=58}, {"Red"=59, "Green"=59, "Blue"=59}, {"Red"=60, "Green"=60, "Blue"=60}, {"Red"=61, "Green"=61, "Blue"=61}, {"Red"=62, "Green"=62, "Blue"=62}, {"Red"=63, "Green"=63, "Blue"=63}, {"Red"=64, "Green"=64, "Blue"=64}, {"Red"=65, "Green"=65, "Blue"=65}, {"Red"=66, "Green"=66, "Blue"=66}, {"Red"=67, "Green"=67, "Blue"=67}, {"Red"=68, "Green"=68, "Blue"=68}, {"Red"=69, "Green"=69, "Blue"=69}, {"Red"=70, "Green"=70, "Blue"=70}, {"Red"=71, "Green"=71, "Blue"=71}, {"Red"=72, "Green"=72, "Blue"=72}, {"Red"=73, "Green"=73, "Blue"=73}, {"Red"=74, "Green"=74, "Blue"=74}, {"Red"=75, "Green"=75, "Blue"=75}, {"Red"=76, "Green"=76, "Blue"=76}, {"Red"=77, "Green"=77, "Blue"=77}, {"Red"=78, "Green"=78, "Blue"=78}, {"Red"=79, "Green"=79, "Blue"=79}, {"Red"=80, "Green"=80, "Blue"=80}, {"Red"=81, "Green"=81, "Blue"=81}, {"Red"=82, "Green"=82, "Blue"=82}, {"Red"=83, "Green"=83, "Blue"=83}, {"Red"=84, "Green"=84, "Blue"=84}, {"Red"=85, "Green"=85, "Blue"=85}, {"Red"=86, "Green"=86, "Blue"=86}, {"Red"=87, "Green"=87, "Blue"=87}, {"Red"=88, "Green"=88, "Blue"=88}, {"Red"=89, "Green"=89, "Blue"=89}, {"Red"=90, "Green"=90, "Blue"=90}, {"Red"=91, "Green"=91, "Blue"=91}, {"Red"=92, "Green"=92, "Blue"=92}, {"Red"=93, "Green"=93, "Blue"=93}, {"Red"=94, "Green"=94, "Blue"=94}, {"Red"=95, "Green"=95, "Blue"=95}, {"Red"=96, "Green"=96, "Blue"=96}, {"Red"=97, "Green"=97, "Blue"=97}, {"Red"=98, "Green"=98, "Blue"=98}, {"Red"=99, "Green"=99, "Blue"=99}, {"Red"=100, "Green"=100, "Blue"=100}, {"Red"=101, "Green"=101, "Blue"=101}, {"Red"=102, "Green"=102, "Blue"=102}, {"Red"=103, "Green"=103, "Blue"=103}, {"Red"=104, "Green"=104, "Blue"=104}, {"Red"=105, "Green"=105, "Blue"=105}, {"Red"=106, "Green"=106, "Blue"=106}, {"Red"=107, "Green"=107, "Blue"=107}, {"Red"=108, "Green"=108, "Blue"=108}, {"Red"=109, "Green"=109, "Blue"=109}, {"Red"=110, "Green"=110, "Blue"=110}, {"Red"=111, "Green"=111, "Blue"=111}, {"Red"=112, "Green"=112, "Blue"=112}, {"Red"=113, "Green"=113, "Blue"=113}, {"Red"=114, "Green"=114, "Blue"=114}, {"Red"=115, "Green"=115, "Blue"=115}, {"Red"=116, "Green"=116, "Blue"=116}, {"Red"=117, "Green"=117, "Blue"=117}, {"Red"=118, "Green"=118, "Blue"=118}, {"Red"=119, "Green"=119, "Blue"=119}, {"Red"=120, "Green"=120, "Blue"=120}, {"Red"=121, "Green"=121, "Blue"=121}, {"Red"=122, "Green"=122, "Blue"=122}, {"Red"=123, "Green"=123, "Blue"=123}, {"Red"=124, "Green"=124, "Blue"=124}, {"Red"=125, "Green"=125, "Blue"=125}, {"Red"=126, "Green"=126, "Blue"=126}, {"Red"=127, "Green"=127, "Blue"=127}, {"Red"=128, "Green"=128, "Blue"=128}, {"Red"=129, "Green"=129, "Blue"=129}, {"Red"=130, "Green"=130, "Blue"=130}, {"Red"=131, "Green"=131, "Blue"=131}, {"Red"=132, "Green"=132, "Blue"=132}, {"Red"=133, "Green"=133, "Blue"=133}, {"Red"=134, "Green"=134, "Blue"=134}, {"Red"=135, "Green"=135, "Blue"=135}, {"Red"=136, "Green"=136, "Blue"=136}, {"Red"=137, "Green"=137, "Blue"=137}, {"Red"=138, "Green"=138, "Blue"=138}, {"Red"=139, "Green"=139, "Blue"=139}, {"Red"=140, "Green"=140, "Blue"=140}, {"Red"=141, "Green"=141, "Blue"=141}, {"Red"=142, "Green"=142, "Blue"=142}, {"Red"=143, "Green"=143, "Blue"=143}, {"Red"=144, "Green"=144, "Blue"=144}, {"Red"=145, "Green"=145, "Blue"=145}, {"Red"=146, "Green"=146, "Blue"=146}, {"Red"=147, "Green"=147, "Blue"=147}, {"Red"=148, "Green"=148, "Blue"=148}, {"Red"=149, "Green"=149, "Blue"=149}, {"Red"=150, "Green"=150, "Blue"=150}, {"Red"=151, "Green"=151, "Blue"=151}, {"Red"=152, "Green"=152, "Blue"=152}, {"Red"=153, "Green"=153, "Blue"=153}, {"Red"=154, "Green"=154, "Blue"=154}, {"Red"=155, "Green"=155, "Blue"=155}, {"Red"=156, "Green"=156, "Blue"=156}, {"Red"=157, "Green"=157, "Blue"=157}, {"Red"=158, "Green"=158, "Blue"=158}, {"Red"=159, "Green"=159, "Blue"=159}, {"Red"=160, "Green"=160, "Blue"=160}, {"Red"=161, "Green"=161, "Blue"=161}, {"Red"=162, "Green"=162, "Blue"=162}, {"Red"=163, "Green"=163, "Blue"=163}, {"Red"=164, "Green"=164, "Blue"=164}, {"Red"=165, "Green"=165, "Blue"=165}, {"Red"=166, "Green"=166, "Blue"=166}, {"Red"=167, "Green"=167, "Blue"=167}, {"Red"=168, "Green"=168, "Blue"=168}, {"Red"=169, "Green"=169, "Blue"=169}, {"Red"=170, "Green"=170, "Blue"=170}, {"Red"=171, "Green"=171, "Blue"=171}, {"Red"=172, "Green"=172, "Blue"=172}, {"Red"=173, "Green"=173, "Blue"=173}, {"Red"=174, "Green"=174, "Blue"=174}, {"Red"=175, "Green"=175, "Blue"=175}, {"Red"=176, "Green"=176, "Blue"=176}, {"Red"=177, "Green"=177, "Blue"=177}, {"Red"=178, "Green"=178, "Blue"=178}, {"Red"=179, "Green"=179, "Blue"=179}, {"Red"=180, "Green"=180, "Blue"=180}, {"Red"=181, "Green"=181, "Blue"=181}, {"Red"=182, "Green"=182, "Blue"=182}, {"Red"=183, "Green"=183, "Blue"=183}, {"Red"=184, "Green"=184, "Blue"=184}, {"Red"=185, "Green"=185, "Blue"=185}, {"Red"=186, "Green"=186, "Blue"=186}, {"Red"=187, "Green"=187, "Blue"=187}, {"Red"=188, "Green"=188, "Blue"=188}, {"Red"=189, "Green"=189, "Blue"=189}, {"Red"=190, "Green"=190, "Blue"=190}, {"Red"=191, "Green"=191, "Blue"=191}, {"Red"=192, "Green"=192, "Blue"=192}, {"Red"=193, "Green"=193, "Blue"=193}, {"Red"=194, "Green"=194, "Blue"=194}, {"Red"=195, "Green"=195, "Blue"=195}, {"Red"=196, "Green"=196, "Blue"=196}, {"Red"=197, "Green"=197, "Blue"=197}, {"Red"=198, "Green"=198, "Blue"=198}, {"Red"=199, "Green"=199, "Blue"=199}, {"Red"=200, "Green"=200, "Blue"=200}, {"Red"=201, "Green"=201, "Blue"=201}, {"Red"=202, "Green"=202, "Blue"=202}, {"Red"=203, "Green"=203, "Blue"=203}, {"Red"=204, "Green"=204, "Blue"=204}, {"Red"=205, "Green"=205, "Blue"=205}, {"Red"=206, "Green"=206, "Blue"=206}, {"Red"=207, "Green"=207, "Blue"=207}, {"Red"=208, "Green"=208, "Blue"=208}, {"Red"=209, "Green"=209, "Blue"=209}, {"Red"=210, "Green"=210, "Blue"=210}, {"Red"=211, "Green"=211, "Blue"=211}, {"Red"=212, "Green"=212, "Blue"=212}, {"Red"=213, "Green"=213, "Blue"=213}, {"Red"=214, "Green"=214, "Blue"=214}, {"Red"=215, "Green"=215, "Blue"=215}, {"Red"=216, "Green"=216, "Blue"=216}, {"Red"=217, "Green"=217, "Blue"=217}, {"Red"=218, "Green"=218, "Blue"=218}, {"Red"=219, "Green"=219, "Blue"=219}, {"Red"=220, "Green"=220, "Blue"=220}, {"Red"=221, "Green"=221, "Blue"=221}, {"Red"=222, "Green"=222, "Blue"=222}, {"Red"=223, "Green"=223, "Blue"=223}, {"Red"=224, "Green"=224, "Blue"=224}, {"Red"=225, "Green"=225, "Blue"=225}, {"Red"=226, "Green"=226, "Blue"=226}, {"Red"=227, "Green"=227, "Blue"=227}, {"Red"=228, "Green"=228, "Blue"=228}, {"Red"=229, "Green"=229, "Blue"=229}, {"Red"=230, "Green"=230, "Blue"=230}, {"Red"=231, "Green"=231, "Blue"=231}, {"Red"=232, "Green"=232, "Blue"=232}, {"Red"=233, "Green"=233, "Blue"=233}, {"Red"=234, "Green"=234, "Blue"=234}, {"Red"=235, "Green"=235, "Blue"=235}, {"Red"=236, "Green"=236, "Blue"=236}, {"Red"=237, "Green"=237, "Blue"=237}, {"Red"=238, "Green"=238, "Blue"=238}, {"Red"=239, "Green"=239, "Blue"=239}, {"Red"=240, "Green"=240, "Blue"=240}, {"Red"=241, "Green"=241, "Blue"=241}, {"Red"=242, "Green"=242, "Blue"=242}, {"Red"=243, "Green"=243, "Blue"=243}, {"Red"=244, "Green"=244, "Blue"=244}, {"Red"=245, "Green"=245, "Blue"=245}, {"Red"=246, "Green"=246, "Blue"=246}, {"Red"=247, "Green"=247, "Blue"=247}, {"Red"=248, "Green"=248, "Blue"=248}, {"Red"=249, "Green"=249, "Blue"=249}, {"Red"=250, "Green"=250, "Blue"=250}, {"Red"=251, "Green"=251, "Blue"=251}, {"Red"=252, "Green"=252, "Blue"=252}, {"Red"=253, "Green"=253, "Blue"=253}, {"Red"=254, "Green"=254, "Blue"=254}, {"Red"=255, "Green"=0, "Blue"=0}] ("Color Palette") cluster{"Red":u8, "Green":u8, "Blue":u8}[] [{"Red"=0, "Green"=0, "Blue"=0}, {"Red"=1, "Green"=1, "Blue"=1}, {"Red"=2, "Green"=2, "Blue"=2}, {"Red"=3, "Green"=3, "Blue"=3}, {"Red"=4, "Green"=4, "Blue"=4}, {"Red"=5, "Green"=5, "Blue"=5}, {"Red"=6, "Green"=6, "Blue"=6}, {"Red"=7, "Green"=7, "Blue"=7}, {"Red"=8, "Green"=8, "Blue"=8}, {"Red"=9, "Green"=9, "Blue"=9}, {"Red"=10, "Green"=10, "Blue"=10}, {"Red"=11, "Green"=11, "Blue"=11}, {"Red"=12, "Green"=12, "Blue"=12}, {"Red"=13, "Green"=13, "Blue"=13}, {"Red"=14, "Green"=14, "Blue"=14}, {"Red"=15, "Green"=15, "Blue"=15}, {"Red"=16, "Green"=16, "Blue"=16}, {"Red"=17, "Green"=17, "Blue"=17}, {"Red"=18, "Green"=18, "Blue"=18}, {"Red"=19, "Green"=19, "Blue"=19}, {"Red"=20, "Green"=20, "Blue"=20}, {"Red"=21, "Green"=21, "Blue"=21}, {"Red"=22, "Green"=22, "Blue"=22}, {"Red"=23, "Green"=23, "Blue"=23}, {"Red"=24, "Green"=24, "Blue"=24}, {"Red"=25, "Green"=25, "Blue"=25}, {"Red"=26, "Green"=26, "Blue"=26}, {"Red"=27, "Green"=27, "Blue"=27}, {"Red"=28, "Green"=28, "Blue"=28}, {"Red"=29, "Green"=29, "Blue"=29}, {"Red"=30, "Green"=30, "Blue"=30}, {"Red"=31, "Green"=31, "Blue"=31}, {"Red"=32, "Green"=32, "Blue"=32}, {"Red"=33, "Green"=33, "Blue"=33}, {"Red"=34, "Green"=34, "Blue"=34}, {"Red"=35, "Green"=35, "Blue"=35}, {"Red"=36, "Green"=36, "Blue"=36}, {"Red"=37, "Green"=37, "Blue"=37}, {"Red"=38, "Green"=38, "Blue"=38}, {"Red"=39, "Green"=39, "Blue"=39}, {"Red"=40, "Green"=40, "Blue"=40}, {"Red"=41, "Green"=41, "Blue"=41}, {"Red"=42, "Green"=42, "Blue"=42}, {"Red"=43, "Green"=43, "Blue"=43}, {"Red"=44, "Green"=44, "Blue"=44}, {"Red"=45, "Green"=45, "Blue"=45}, {"Red"=46, "Green"=46, "Blue"=46}, {"Red"=47, "Green"=47, "Blue"=47}, {"Red"=48, "Green"=48, "Blue"=48}, {"Red"=49, "Green"=49, "Blue"=49}, {"Red"=50, "Green"=50, "Blue"=50}, {"Red"=51, "Green"=51, "Blue"=51}, {"Red"=52, "Green"=52, "Blue"=52}, {"Red"=53, "Green"=53, "Blue"=53}, {"Red"=54, "Green"=54, "Blue"=54}, {"Red"=55, "Green"=55, "Blue"=55}, {"Red"=56, "Green"=56, "Blue"=56}, {"Red"=57, "Green"=57, "Blue"=57}, {"Red"=58, "Green"=58, "Blue"=58}, {"Red"=59, "Green"=59, "Blue"=59}, {"Red"=60, "Green"=60, "Blue"=60}, {"Red"=61, "Green"=61, "Blue"=61}, {"Red"=62, "Green"=62, "Blue"=62}, {"Red"=63, "Green"=63, "Blue"=63}, {"Red"=64, "Green"=64, "Blue"=64}, {"Red"=65, "Green"=65, "Blue"=65}, {"Red"=66, "Green"=66, "Blue"=66}, {"Red"=67, "Green"=67, "Blue"=67}, {"Red"=68, "Green"=68, "Blue"=68}, {"Red"=69, "Green"=69, "Blue"=69}, {"Red"=70, "Green"=70, "Blue"=70}, {"Red"=71, "Green"=71, "Blue"=71}, {"Red"=72, "Green"=72, "Blue"=72}, {"Red"=73, "Green"=73, "Blue"=73}, {"Red"=74, "Green"=74, "Blue"=74}, {"Red"=75, "Green"=75, "Blue"=75}, {"Red"=76, "Green"=76, "Blue"=76}, {"Red"=77, "Green"=77, "Blue"=77}, {"Red"=78, "Green"=78, "Blue"=78}, {"Red"=79, "Green"=79, "Blue"=79}, {"Red"=80, "Green"=80, "Blue"=80}, {"Red"=81, "Green"=81, "Blue"=81}, {"Red"=82, "Green"=82, "Blue"=82}, {"Red"=83, "Green"=83, "Blue"=83}, {"Red"=84, "Green"=84, "Blue"=84}, {"Red"=85, "Green"=85, "Blue"=85}, {"Red"=86, "Green"=86, "Blue"=86}, {"Red"=87, "Green"=87, "Blue"=87}, {"Red"=88, "Green"=88, "Blue"=88}, {"Red"=89, "Green"=89, "Blue"=89}, {"Red"=90, "Green"=90, "Blue"=90}, {"Red"=91, "Green"=91, "Blue"=91}, {"Red"=92, "Green"=92, "Blue"=92}, {"Red"=93, "Green"=93, "Blue"=93}, {"Red"=94, "Green"=94, "Blue"=94}, {"Red"=95, "Green"=95, "Blue"=95}, {"Red"=96, "Green"=96, "Blue"=96}, {"Red"=97, "Green"=97, "Blue"=97}, {"Red"=98, "Green"=98, "Blue"=98}, {"Red"=99, "Green"=99, "Blue"=99}, {"Red"=100, "Green"=100, "Blue"=100}, {"Red"=101, "Green"=101, "Blue"=101}, {"Red"=102, "Green"=102, "Blue"=102}, {"Red"=103, "Green"=103, "Blue"=103}, {"Red"=104, "Green"=104, "Blue"=104}, {"Red"=105, "Green"=105, "Blue"=105}, {"Red"=106, "Green"=106, "Blue"=106}, {"Red"=107, "Green"=107, "Blue"=107}, {"Red"=108, "Green"=108, "Blue"=108}, {"Red"=109, "Green"=109, "Blue"=109}, {"Red"=110, "Green"=110, "Blue"=110}, {"Red"=111, "Green"=111, "Blue"=111}, {"Red"=112, "Green"=112, "Blue"=112}, {"Red"=113, "Green"=113, "Blue"=113}, {"Red"=114, "Green"=114, "Blue"=114}, {"Red"=115, "Green"=115, "Blue"=115}, {"Red"=116, "Green"=116, "Blue"=116}, {"Red"=117, "Green"=117, "Blue"=117}, {"Red"=118, "Green"=118, "Blue"=118}, {"Red"=119, "Green"=119, "Blue"=119}, {"Red"=120, "Green"=120, "Blue"=120}, {"Red"=121, "Green"=121, "Blue"=121}, {"Red"=122, "Green"=122, "Blue"=122}, {"Red"=123, "Green"=123, "Blue"=123}, {"Red"=124, "Green"=124, "Blue"=124}, {"Red"=125, "Green"=125, "Blue"=125}, {"Red"=126, "Green"=126, "Blue"=126}, {"Red"=127, "Green"=127, "Blue"=127}, {"Red"=128, "Green"=128, "Blue"=128}, {"Red"=129, "Green"=129, "Blue"=129}, {"Red"=130, "Green"=130, "Blue"=130}, {"Red"=131, "Green"=131, "Blue"=131}, {"Red"=132, "Green"=132, "Blue"=132}, {"Red"=133, "Green"=133, "Blue"=133}, {"Red"=134, "Green"=134, "Blue"=134}, {"Red"=135, "Green"=135, "Blue"=135}, {"Red"=136, "Green"=136, "Blue"=136}, {"Red"=137, "Green"=137, "Blue"=137}, {"Red"=138, "Green"=138, "Blue"=138}, {"Red"=139, "Green"=139, "Blue"=139}, {"Red"=140, "Green"=140, "Blue"=140}, {"Red"=141, "Green"=141, "Blue"=141}, {"Red"=142, "Green"=142, "Blue"=142}, {"Red"=143, "Green"=143, "Blue"=143}, {"Red"=144, "Green"=144, "Blue"=144}, {"Red"=145, "Green"=145, "Blue"=145}, {"Red"=146, "Green"=146, "Blue"=146}, {"Red"=147, "Green"=147, "Blue"=147}, {"Red"=148, "Green"=148, "Blue"=148}, {"Red"=149, "Green"=149, "Blue"=149}, {"Red"=150, "Green"=150, "Blue"=150}, {"Red"=151, "Green"=151, "Blue"=151}, {"Red"=152, "Green"=152, "Blue"=152}, {"Red"=153, "Green"=153, "Blue"=153}, {"Red"=154, "Green"=154, "Blue"=154}, {"Red"=155, "Green"=155, "Blue"=155}, {"Red"=156, "Green"=156, "Blue"=156}, {"Red"=157, "Green"=157, "Blue"=157}, {"Red"=158, "Green"=158, "Blue"=158}, {"Red"=159, "Green"=159, "Blue"=159}, {"Red"=160, "Green"=160, "Blue"=160}, {"Red"=161, "Green"=161, "Blue"=161}, {"Red"=162, "Green"=162, "Blue"=162}, {"Red"=163, "Green"=163, "Blue"=163}, {"Red"=164, "Green"=164, "Blue"=164}, {"Red"=165, "Green"=165, "Blue"=165}, {"Red"=166, "Green"=166, "Blue"=166}, {"Red"=167, "Green"=167, "Blue"=167}, {"Red"=168, "Green"=168, "Blue"=168}, {"Red"=169, "Green"=169, "Blue"=169}, {"Red"=170, "Green"=170, "Blue"=170}, {"Red"=171, "Green"=171, "Blue"=171}, {"Red"=172, "Green"=172, "Blue"=172}, {"Red"=173, "Green"=173, "Blue"=173}, {"Red"=174, "Green"=174, "Blue"=174}, {"Red"=175, "Green"=175, "Blue"=175}, {"Red"=176, "Green"=176, "Blue"=176}, {"Red"=177, "Green"=177, "Blue"=177}, {"Red"=178, "Green"=178, "Blue"=178}, {"Red"=179, "Green"=179, "Blue"=179}, {"Red"=180, "Green"=180, "Blue"=180}, {"Red"=181, "Green"=181, "Blue"=181}, {"Red"=182, "Green"=182, "Blue"=182}, {"Red"=183, "Green"=183, "Blue"=183}, {"Red"=184, "Green"=184, "Blue"=184}, {"Red"=185, "Green"=185, "Blue"=185}, {"Red"=186, "Green"=186, "Blue"=186}, {"Red"=187, "Green"=187, "Blue"=187}, {"Red"=188, "Green"=188, "Blue"=188}, {"Red"=189, "Green"=189, "Blue"=189}, {"Red"=190, "Green"=190, "Blue"=190}, {"Red"=191, "Green"=191, "Blue"=191}, {"Red"=192, "Green"=192, "Blue"=192}, {"Red"=193, "Green"=193, "Blue"=193}, {"Red"=194, "Green"=194, "Blue"=194}, {"Red"=195, "Green"=195, "Blue"=195}, {"Red"=196, "Green"=196, "Blue"=196}, {"Red"=197, "Green"=197, "Blue"=197}, {"Red"=198, "Green"=198, "Blue"=198}, {"Red"=199, "Green"=199, "Blue"=199}, {"Red"=200, "Green"=200, "Blue"=200}, {"Red"=201, "Green"=201, "Blue"=201}, {"Red"=202, "Green"=202, "Blue"=202}, {"Red"=203, "Green"=203, "Blue"=203}, {"Red"=204, "Green"=204, "Blue"=204}, {"Red"=205, "Green"=205, "Blue"=205}, {"Red"=206, "Green"=206, "Blue"=206}, {"Red"=207, "Green"=207, "Blue"=207}, {"Red"=208, "Green"=208, "Blue"=208}, {"Red"=209, "Green"=209, "Blue"=209}, {"Red"=210, "Green"=210, "Blue"=210}, {"Red"=211, "Green"=211, "Blue"=211}, {"Red"=212, "Green"=212, "Blue"=212}, {"Red"=213, "Green"=213, "Blue"=213}, {"Red"=214, "Green"=214, "Blue"=214}, {"Red"=215, "Green"=215, "Blue"=215}, {"Red"=216, "Green"=216, "Blue"=216}, {"Red"=217, "Green"=217, "Blue"=217}, {"Red"=218, "Green"=218, "Blue"=218}, {"Red"=219, "Green"=219, "Blue"=219}, {"Red"=220, "Green"=220, "Blue"=220}, {"Red"=221, "Green"=221, "Blue"=221}, {"Red"=222, "Green"=222, "Blue"=222}, {"Red"=223, "Green"=223, "Blue"=223}, {"Red"=224, "Green"=224, "Blue"=224}, {"Red"=225, "Green"=225, "Blue"=225}, {"Red"=226, "Green"=226, "Blue"=226}, {"Red"=227, "Green"=227, "Blue"=227}, {"Red"=228, "Green"=228, "Blue"=228}, {"Red"=229, "Green"=229, "Blue"=229}, {"Red"=230, "Green"=230, "Blue"=230}, {"Red"=231, "Green"=231, "Blue"=231}, {"Red"=232, "Green"=232, "Blue"=232}, {"Red"=233, "Green"=233, "Blue"=233}, {"Red"=234, "Green"=234, "Blue"=234}, {"Red"=235, "Green"=235, "Blue"=235}, {"Red"=236, "Green"=236, "Blue"=236}, {"Red"=237, "Green"=237, "Blue"=237}, {"Red"=238, "Green"=238, "Blue"=238}, {"Red"=239, "Green"=239, "Blue"=239}, {"Red"=240, "Green"=240, "Blue"=240}, {"Red"=241, "Green"=241, "Blue"=241}, {"Red"=242, "Green"=242, "Blue"=242}, {"Red"=243, "Green"=243, "Blue"=243}, {"Red"=244, "Green"=244, "Blue"=244}, {"Red"=245, "Green"=245, "Blue"=245}, {"Red"=246, "Green"=246, "Blue"=246}, {"Red"=247, "Green"=247, "Blue"=247}, {"Red"=248, "Green"=248, "Blue"=248}, {"Red"=249, "Green"=249, "Blue"=249}, {"Red"=250, "Green"=250, "Blue"=250}, {"Red"=251, "Green"=251, "Blue"=251}, {"Red"=252, "Green"=252, "Blue"=252}, {"Red"=253, "Green"=253, "Blue"=253}, {"Red"=254, "Green"=254, "Blue"=254}, {"Red"=255, "Green"=255, "Blue"=255}] ("Color Palette")] -> w94
              frame "high clipping red" {
              }
              frame "low clipping blue" {
              }
              frame "high and low clipping" {
              }
              frame "standard" {
              }
            }
            n61 = call-poly "GFGpolyGet.vi"() -> ("error out"=w102:errorcluster, "DisplayRefsOut(generic class)"=w101:T13)  [unwired: 10 in]
            n62 = Cluster To Array(cluster=w101) -> (array=w99:refnum<vi>[])
            n63 = for {
              tunnel: w99 -> [w109] mode=indexing
              tunnel: w94 -> [w113]
              tunnel: w98 -> [w112]
              tunnel: w102 -> [w111]
              tunnel: [w110] -> _
              tunnel: w100 -> [w107]
              n64 = To More Specific Class(target class=w107, reference=w109) -> (specific class reference=w108:refnum<vi>)  [unwired: 1 in, 1 out]
              n65 = property class="ImageControl"(reference=w108, error in=w111, "User Palette"=w113, "Palette Type"=w112) -> (error out=w110:errorcluster)  [unwired: 1 out]
            }
          }
          frame "display.queue.to.fp.display_MD.completed", "galvo.scan.engine_MD.completed", "image.queue.to.disk.and.display.queue_MD.completed", "raw.queue.to.image.queue_MD.completed" {
            n66 = for {
              N: 1 -> [_]
              shift-right: [w128] -> _
              shift-left: _ -> [w130]
              tunnel: [w129] -> w121
              n67 = Tick Count (ms)() -> (millisecond timer value=w128:u32)
              n68 = Subtract(x=w128, y=w130) -> (x-y=w129:u32)
            }
            n69 = Greater?(x=u32 500 ("y"), y=w121) -> (0:w118:bool)
            n70 = local read "String"() -> (w117:string)
            n71 = Select(t=w117, s=w118, f="") -> (s? t:f=w119:string)
            n72 = Concatenate Strings(w119, "\r\n", w115) -> (w126:string)
            n73 = for {
              tunnel: w126 -> [w137]
              tunnel: string[] ["galvo.scan.engine_MD.completed", "raw.queue.to.image.queue_MD.completed", "image.queue.to.disk.and.display.queue_MD.completed", "display.queue.to.fp.display_MD.completed"] ("appended array") -> [w136] mode=indexing
              shift-right: [w132] -> w123
              shift-left: i16 0 -> [w131]
              n74 = Match Pattern(string=w137, regular expression=w136) -> (offset past match=w135:i32)  [unwired: 1 in, 3 out]
              n75 = Greater Or Equal To 0?(x=w135) -> (x >= 0?=w134:bool)
              n76 = Boolean To (0,1)(Boolean=w134) -> (0, 1=w133:i16)
              n77 = Add(x=w133, y=w131) -> (x+y=w132:i16)
            }
            n78 = local write "String"(w126) -> ()
            n79 = disable-structure shown="Enabled" {
              disable-tunnel: w123 -> [w139 _]
              frame Enabled {
                n80 = Equal?(x=w139, y=4) -> (x = y?=w138:bool)
                n81 = case shown="True" w138 {
                  selector: w138 -> [_ w141]
                  frame False {
                  }
                  frame True {
                    n82 = call "GFG_core.vi"("Variable Name in"="flystop", "Variant in"=FALSE ("x = y?"), "Action"=enum16{"Init", "Set", "Get"}."Set") -> ()  [unwired: 10 in, 7 out]
                    n83 = local write "String"("") -> ()
                    "ready for flystart?" <- w141
                  }
                }
              }
              frame Disabled {
              }
            }
          }
          frame "ROTATE", "Start.Delay", "fill.fraction", "max.field.of.view", "nomin.x.pixels", "pixel.dwell.time.in.sec", "rotate.enable", "voltage.for.max.field.of.view", "x.bidirectional", "x.pixel.sz", "x.volt.offset", "y.bidirectional", "y.pixel.sz", "y.pixels", "y.volt.offset" {
            n84 = for {
              N: 1 -> [_]
              tunnel: [w159] -> w148 mode=indexing
              shift-right: [w155] -> _
              shift-left: _ -> [w157]
              tunnel: [w154] -> w146
              n85 = Tick Count (ms)() -> (millisecond timer value=w155:u32)
              n86 = Subtract(x=w155, y=w157) -> (x-y=w158:u32)
              n87 = Greater?(x=w158, y=u32 500) -> (0:w154:bool)
              n88 = case shown="True" w154 {
                tunnel: [_ w162] -> w159
                frame False {
                }
                frame True {
                  n89 = call-poly "GFGpolyGet.vi"("Variable Name in"="FOCUS") -> ("Boolean"=w160:bool)  [unwired: 10 in]
                  n90 = case shown="True" w160 {
                    frame False {
                    }
                    frame True {
                      n91 = call "kill task and queues for flystart.vi"() -> ()  [unwired: 12 in]
                    }
                  }
                  n92 = call "GFG_core.vi"("Variable Name in"="flystop", "Variant in"=w160, "Action"=enum16{"Init", "Set", "Get"}."Set") -> ("error out"=w162:errorcluster)  [unwired: 10 in, 6 out]
                  n93 = Wait (ms)(milliseconds to wait=u32 50) -> ()  [unwired: 1 out]
                }
              }
            }
            n94 = case shown="\"False\", Default" w153 {
              tunnel: w152 -> [_ w176 _ _]
              tunnel: w151 -> [_ _ w199 _]
              tunnel: w150 -> [_ _ _ w206]
              tunnel: w148 -> [_ _ _ _]
              tunnel: w146 -> [w166 _ _ _]
              frame "False", Default {
                n95 = case shown="True" w166 {
                  frame False {
                  }
                  frame True {
                    n96 = call "GFG refresh all variables.vi"("All Variable Names"=string[] ["ZOOM"]) -> ()  [unwired: 11 in]
                  }
                }
              }
              frame "x.bidirectional" {
                n97 = Variant To Data(type=TRUE, Variant=w176) -> (data=w169:bool)  [unwired: 1 in, 1 out]
                n98 = call-poly "GFGpolyGet.vi"("Variable Name in"="speed mode") -> ("output cluster"=w173:T12)  [unwired: 9 in, 1 out]
                n99 = call "GFG_core.vi"("Variable Name in"="scan mode main settings") -> ("Variant Out"=w179:variant)  [unwired: 12 in, 6 out]
                n100 = Unbundle By Name(w173) -> ("RingRef"=w172:refnum<vi>)
                n101 = Variant To Data(type=scan_mode_main_settings_tab."2D line scan" ("scan mode main settings"), Variant=w179) -> (data=w177:T2)  [unwired: 1 in, 1 out]
                n102 = case shown="\"2D frame\", Default" w177 {
                  tunnel: w169 -> [w186 _]
                  frame "2D frame", Default {
                    n103 = call-poly "GFGpolyGet.vi"("Variable Name in"="MAIN Image panels ") -> ("output cluster"=w182:T12)  [unwired: 9 in, 1 out]
                    n104 = call "GFG_core.vi"("Variable Name in"="fill.fraction.bidi") -> ("Variant Out"=w188:variant)  [unwired: 12 in, 6 out]
                    n105 = Unbundle By Name(w182) -> ("TabControlRef"=w184:refnum<vi>)
                    n106 = call "GFG_core.vi"("Variable Name in"="fill.fraction.unidi") -> ("Variant Out"=w189:variant)  [unwired: 12 in, 6 out]
                    n107 = Select(t=w188, s=w186, f=w189) -> (s? t:f=w187:variant)
                    n108 = call "GFG_core.vi"("Variable Name in"="fill.fraction", "Variant in"=w187, "Action"=enum16{"Init", "Set", "Get"}."Set") -> ()  [unwired: 10 in, 7 out]
                    n109 = property class="TabCtl"(reference=w184, "Tabs Visible?"=TRUE) -> ()  [unwired: 1 in, 2 out]
                    n110 = call "GFG refresh all variables.vi"("All Variable Names"=string[] ["pixel resolution"]) -> ()  [unwired: 11 in]
                  }
                  frame "2D line scan" {
                    n111 = call "GFG_core.vi"("Variable Name in"="fill.fraction.line", "Action"=enum16{"Init", "Set", "Get"}."Get") -> ("Variant Out"=w194:variant)  [unwired: 11 in, 6 out]
                    n112 = call "GFG_core.vi"("Variable Name in"="fill.fraction", "Variant in"=w194, "Action"=enum16{"Init", "Set", "Get"}."Set") -> ()  [unwired: 10 in, 7 out]
                  }
                }
                n113 = Select(t=i32[] [] ("Disabled Items []"), s=w169, f=i32[] [0, 1] ("Disabled Items []")) -> (s? t:f=w168:i32[])
                n114 = property class="Ring"(reference=w172, "Disabled Items []"=w168) -> ()  [unwired: 1 in, 2 out]
              }
              frame "pixel.dwell.time.in.sec." {
                n115 = call "GFG_core.vi"("Variable Name in"="scan mode main settings") -> ("Variant Out"=w202:variant)  [unwired: 12 in, 6 out]
                n116 = Variant To Data(type=scan_mode_main_settings_tab."2D line scan" ("scan mode main settings"), Variant=w202) -> (data=w200:T2)  [unwired: 1 in, 1 out]
                n117 = case shown="\"2D frame\", Default" w200 {
                  tunnel: [5 w205] -> _
                  tunnel: w199 -> [_ w205]
                  frame "2D frame", Default {
                  }
                  frame "2D line scan" {
                  }
                }
              }
              frame "fill.fraction" {
                n118 = call "getVIname.vi"() -> ("VI name"=w207:string)  [unwired: 19 in]
                n119 = Not Equal?(x=w207, y=w206) -> (x != y?=w208:bool)
                n120 = case shown="True" w208 {
                  frame False {
                  }
                  frame True {
                    n121 = call "GFG_core.vi"("Variable Name in"="x.bidirectional") -> ("Variant Out"=w215:variant)  [unwired: 12 in, 6 out]
                    n122 = call "GFG_core.vi"("Variable Name in"="scan mode main settings") -> ("Variant Out"=w212:variant)  [unwired: 12 in, 6 out]
                    n123 = Variant To Data(type=TRUE, Variant=w215) -> (data=w214:bool)  [unwired: 1 in, 1 out]
                    n124 = Variant To Data(type=scan_mode_main_settings_tab."2D line scan" ("scan mode main settings"), Variant=w212) -> (data=w209:T2)  [unwired: 1 in, 1 out]
                    n125 = case shown="\"2D frame\", Default" w209 {
                      tunnel: w214 -> [w217 _]
                      frame "2D frame", Default {
                        n126 = case shown="False" w217 {
                          frame False {
                            n127 = call "GFG_core.vi"("Variable Name in"="fill.fraction") -> ("Variant Out"=w218:variant)  [unwired: 12 in, 6 out]
                            n128 = call "GFG_core.vi"("Variable Name in"="fill.fraction.unidi", "Variant in"=w218, "Action"=enum16{"Init", "Set", "Get"}."Set") -> ()  [unwired: 10 in, 7 out]
                          }
                          frame True {
                            n129 = call "GFG_core.vi"("Variable Name in"="fill.fraction") -> ("Variant Out"=w222:variant)  [unwired: 12 in, 6 out]
                            n130 = call "GFG_core.vi"("Variable Name in"="fill.fraction.bidi", "Variant in"=w222, "Action"=enum16{"Init", "Set", "Get"}."Set") -> ()  [unwired: 10 in, 7 out]
                          }
                        }
                      }
                      frame "2D line scan" {
                      }
                    }
                  }
                }
              }
            }
          }
          frame "no..of.frames.to.acquire" {
            n131 = Variant To Data(type=0.0, Variant=w233) -> (data=w227:dbl)  [unwired: 1 in, 1 out]
            n132 = call-poly "GFGpolyGet.vi"("Variable Name in"="frame count") -> ("output cluster"=w235:T12)  [unwired: 9 in, 1 out]
            n133 = call "GFG_core.vi"("Variable Name in"="scan mode main settings") -> ("Variant Out"=w229:variant)  [unwired: 12 in, 6 out]
            n134 = Unbundle By Name(w235) -> ("SlideRef"=w234:refnum<vi>)
            n135 = Variant To Data(type=scan_mode_main_settings_tab."2D line scan" ("scan mode main settings"), Variant=w229) -> (data=w226:T2)  [unwired: 1 in, 1 out]
            n136 = property class="Slide"(reference=w234, "Scale.Maximum"=w227) -> ()  [unwired: 1 in, 2 out]
            n137 = case shown="\"2D frame\", Default" w226 {
              tunnel: w227 -> [w237 _]
              frame "2D frame", Default {
                n138 = call "GFG_core.vi"("Variable Name in"="no.of.frames.for.frame.scan", "Variant in"=w237, "Action"=enum16{"Init", "Set", "Get"}."Set") -> ()  [unwired: 10 in, 7 out]
              }
              frame "2D line scan" {
              }
            }
          }
          frame "reset.zoom" {
            n139 = call-poly "GFGpolyGet.vi"() -> ("DisplayRefsOut(generic class)"=w245:T13)  [unwired: 10 in, 1 out]
            n140 = call-poly "GFGpolyGet.vi"() -> ("Image Refs Out"=w244:T15)  [unwired: 10 in, 1 out]
            n141 = Cluster To Array(cluster=w245) -> (array=w243:refnum<vi>[])
            n142 = Cluster To Array(cluster=w244) -> (array=w242:T14[])
            n143 = call "set initial zoom.vi"("reset?"=TRUE, "Image Refs In"=w242, "DisplayRefsIn(generic class)"=w243) -> ()  [unwired: 9 in]
          }
          frame "ZOOM", "pixel.resolution", "speed.mode" {
            n144 = for {
              N: 1 -> [_]
              tunnel: [w257] -> w246 mode=indexing
              shift-right: [w252] -> _
              shift-left: _ -> [w255]
              n145 = Tick Count (ms)() -> (millisecond timer value=w252:u32)
              n146 = Subtract(x=w252, y=w255) -> (x-y=w256:u32)
              n147 = Greater?(x=w256, y=u32 500) -> (0:w253:bool)
              n148 = case shown="True" w253 {
                tunnel: [_ w260] -> w257
                frame False {
                }
                frame True {
                  n149 = call-poly "GFGpolyGet.vi"("Variable Name in"="FOCUS") -> ("Boolean"=w258:bool)  [unwired: 10 in]
                  n150 = case shown="True" w258 {
                    frame False {
                    }
                    frame True {
                      n151 = call "kill task and queues for flystart.vi"() -> ()  [unwired: 12 in]
                    }
                  }
                  n152 = call "GFG_core.vi"("Variable Name in"="flystop", "Variant in"=w258, "Action"=enum16{"Init", "Set", "Get"}."Set") -> ("error out"=w260:errorcluster)  [unwired: 10 in, 6 out]
                  n153 = Wait (ms)(milliseconds to wait=u32 50) -> ()  [unwired: 1 out]
                }
              }
            }
            n154 = case shown="\"ZOOM\", Default" w249 {
              tunnel: w251 -> [_ w270]
              tunnel: [w264 w268] -> w250
              tunnel: w246 -> [_ _]
              frame "ZOOM", Default {
                n155 = call "GFG_core.vi"("Variable Name in"="pixel.resolution") -> ("Variant Out"=w266:variant)  [unwired: 12 in, 6 out]
                n156 = Variant To Data(type=pixel_resolution_enum."   128 x 128" ("pixel resolution"), Variant=w266) -> (data=w264:T3)  [unwired: 1 in, 1 out]
              }
              frame "pixel.resolution" {
                n157 = Variant To Data(type=pixel_resolution_enum."   128 x 128" ("pixel resolution"), Variant=w270) -> (data=w268:T3)  [unwired: 1 in, 1 out]
              }
            }
            n158 = case shown="Default" w250 {
              selector: w250 -> [_ w292]
              frame "   arbitrary" {
                w273 = "nomin.x.pixels" ("Variable Name in")
                n159 = call-poly "GFGpolyGet.vi"("Variable Name in"="ZOOM") -> ("output cluster"=w278:T12)  [unwired: 9 in, 1 out]
                n160 = call-poly "GFGpolyGet.vi"("Variable Name in"="speed.mode") -> ("output cluster"=w283:T12)  [unwired: 9 in, 1 out]
                n161 = Build Array("nomin.x.pixels" ("Variable Name in"), "y.pixel.sz" ("Variable Name in"), "x.pixel.sz" ("Variable Name in"), "pixel.dwell.time.in.sec" ("Variable Name in")) -> (w284:string[])
                n162 = Unbundle By Name(w278) -> ("SlideRef"=w280:refnum<vi>)
                n163 = Unbundle By Name(w283) -> ("RingRef"=w281:refnum<vi>)
                n164 = property class="Slide"(reference=w280, "DisabledEnum"=T4."Disabled and Grayed Out" ("Disabled")) -> ()  [unwired: 1 in, 2 out]
                n165 = for {
                  tunnel: w284 -> [w291] mode=indexing
                  n166 = call-poly "GFGpolyGet.vi"("Variable Name in"=w291) -> ("output cluster"=w290:T12)  [unwired: 9 in, 1 out]
                  n167 = Unbundle By Name(w290) -> ("DigitalRef"=w288:refnum<vi>)
                  n168 = property class="DigNum"(reference=w288, "DisabledEnum"=T4."Enabled" ("Disabled")) -> ()  [unwired: 1 in, 2 out]
                }
                n169 = property class="Ring"(reference=w281, "DisabledEnum"=T4."Disabled and Grayed Out" ("Disabled")) -> ()  [unwired: 1 in, 2 out]
                n170 = call "GFG_core.vi"("Variable Name in"=w273, "Action"=enum16{"Init", "Set", "Get"}."Get") -> ("Variant Out"=w272:variant)  [unwired: 11 in, 6 out]
                n171 = call "GFG_core.vi"("Variable Name in"=w273, "Variant in"=w272, "Action"=enum16{"Init", "Set", "Get"}."Set") -> ()  [unwired: 10 in, 7 out]
              }
              frame Default {
                w321 = T16 0 items=["high-speed scan", "standard scan", "long exposure"] ("speed mode")
                n172 = Build Array("nomin.x.pixels" ("Variable Name in"), "y.pixel.sz" ("Variable Name in"), "x.pixel.sz" ("Variable Name in"), "pixel.dwell.time.in.sec" ("Variable Name in")) -> (w331:string[])
                n173 = call "GFG_core.vi"("Variable Name in"="speed.mode") -> ("Variant Out"=w320:variant)  [unwired: 12 in, 6 out]
                n174 = for {
                  tunnel: w331 -> [w365] mode=indexing
                  n175 = call-poly "GFGpolyGet.vi"("Variable Name in"=w365) -> ("output cluster"=w364:T12)  [unwired: 9 in, 1 out]
                  n176 = Unbundle By Name(w364) -> ("DigitalRef"=w362:refnum<vi>)
                  n177 = property class="DigNum"(reference=w362, "DisabledEnum"=T4."Disabled and Grayed Out" ("Disabled")) -> (error out=→"error out 2":errorcluster)  [unwired: 1 in, 1 out]
                }
                n178 = Variant To Data(type=w321, Variant=w320) -> (data=w296:T16)  [unwired: 1 in, 1 out]
                n179 = case shown="\"   128 x 128\", Default" w292 {
                  tunnel: [128 256 256 512 512 512 512 1024 1024] -> w294
                  tunnel: [128 128 256 256 128 64 512 512 1024] -> w293
                  frame "   128 x 128", Default {
                  }
                  frame "   256 x 128" {
                  }
                  frame "   256 x 256" {
                  }
                  frame "   512 x 256" {
                  }
                  frame "   512 x 128" {
                  }
                  frame "   512 x  64" {
                  }
                  frame "   512 x 512" {
                  }
                  frame "  1024 x 512" {
                  }
                  frame "  1024 x 1024" {
                  }
                }
                n180 = case shown="0, Default" w296 {
                  tunnel: [1e-06 2e-06 4e-06 8e-06] -> w297
                  frame 0, Default {
                  }
                  frame 1 {
                  }
                  frame 2 {
                  }
                  frame 3 {
                  }
                }
                n181 = call "GFG_core.vi"("Variable Name in"="pixel.dwell.time.in.sec", "Variant in"=w297, "Action"=enum16{"Init", "Set", "Get"}."Set") -> ()  [unwired: 10 in, 7 out]
                n182 = call-poly "GFGpolyGet.vi"("Variable Name in"="max.field.of.view") -> ("Numeric"=w316:dbl)  [unwired: 9 in, 1 out]
                n183 = call "GFG_core.vi"("Variable Name in"="y.pixels", "Variant in"=w293, "Action"=enum16{"Init", "Set", "Get"}."Set") -> ()  [unwired: 10 in, 7 out]
                n184 = call-poly "GFGpolyGet.vi"("Variable Name in"="ZOOM") -> ("Numeric"=w315:dbl)  [unwired: 9 in, 1 out]
                n185 = call "GFG_core.vi"("Variable Name in"="nomin.x.pixels", "Variant in"=w294, "Action"=enum16{"Init", "Set", "Get"}."Set") -> ()  [unwired: 10 in, 7 out]
                n186 = Divide(x=w316, y=w315) -> (x/y=w303:dbl)
                n187 = call-poly "GFGpolyGet.vi"("Variable Name in"="fill.fraction") -> ("Numeric"=w309:dbl)  [unwired: 9 in, 1 out]
                n188 = Build Array(w294, w293) -> (w301:i32[])
                n189 = Divide(x=w309, y=100.0) -> (x/y=w307:dbl)
                n190 = call-poly "GFGpolyGet.vi"("Variable Name in"="ZOOM") -> ("output cluster"=w324:T12)  [unwired: 9 in, 1 out]
                n191 = call-poly "GFGpolyGet.vi"("Variable Name in"="speed.mode") -> ("output cluster"=w329:T12)  [unwired: 9 in, 1 out]
                n192 = Divide(x=w294, y=w307) -> (x/y=w304:dbl)
                n193 = Unbundle By Name(w324) -> ("SlideRef"=w326:refnum<vi>)
                n194 = Unbundle By Name(w329) -> ("RingRef"=w327:refnum<vi>)
                n195 = Array Max & Min(array=w301) -> (max value=w300:i32)  [unwired: 3 out]
                n196 = call "GFG_core.vi"("Variable Name in"="x.pixels", "Variant in"=w304, "Action"=enum16{"Init", "Set", "Get"}."Set") -> ()  [unwired: 10 in, 7 out]
                n197 = property class="Slide"(reference=w326, "DisabledEnum"=T4."Enabled" ("Disabled")) -> ()  [unwired: 1 in, 2 out]
                n198 = Divide(x=w303, y=w300) -> (x/y=w302:dbl)
                n199 = property class="Ring"(reference=w327, "DisabledEnum"=T4."Enabled" ("Disabled")) -> (error out=→"error out":errorcluster)  [unwired: 1 in, 1 out]
                n200 = call "GFG_core.vi"("Variable Name in"="x.pixel.sz", "Variant in"=w302, "Action"=enum16{"Init", "Set", "Get"}."Set") -> ()  [unwired: 10 in, 7 out]
                n201 = call "GFG_core.vi"("Variable Name in"="y.pixel.sz", "Variant in"=w302, "Action"=enum16{"Init", "Set", "Get"}."Set") -> ()  [unwired: 10 in, 7 out]
              }
            }
          }
          frame "piezo.mode" {
            n202 = call-poly "GFGpolyGet.vi"("Variable Name in"="frames.per.z.cycle") -> ("output cluster"=w374:T12)  [unwired: 9 in, 1 out]
            n203 = call-poly "GFGpolyGet.vi"("Variable Name in"="piezo.mode") -> ("Boolean"=w368:bool)  [unwired: 10 in]
            n204 = Unbundle By Name(w374) -> ("DigitalRef"=w373:refnum<vi>)
            n205 = Select(t=T6 {"Minimum"=3.0, "Maximum"=101.0, "Increment"=2.0} ("Data Entry Limits"), s=w368, f=T6 {"Minimum"=4.0, "Maximum"=100.0, "Increment"=2.0} ("Data Entry Limits")) -> (s? t:f=w369:T6)
            n206 = property class="DigNum"(reference=w373, "Data Range"=w369, "OutOfRngAction"=T5 {"Out of Range Action Minimum"=1, "Out of Range Action Maximum"=1, "Out of Range Action Increment"=1} ("Response to Value Outside Limits")) -> ()  [unwired: 1 in, 2 out]
          }
          frame "scan.mode.main.settings" {
            n207 = Variant To Data(type=scan_mode_main_settings_tab."2D frame" ("scan mode main settings"), Variant=w380) -> (data=w378:T2)  [unwired: 1 in, 1 out]
            n208 = case shown="\"Z Stack\"" w378 {
              tunnel: w377 -> [w399 w406 w413]
              tunnel: [w399 w406 w413] -> w376
              frame "2D frame", Default {
                n209 = call "GFG refresh all variables.vi"("All Variable Names"=string[] ["pixel resolution", "x.bidirectional"]) -> ()  [unwired: 11 in]
                n210 = call "GFG_core.vi"("Variable Name in"="no..of.frames.for.frame.scan", "Action"=enum16{"Init", "Set", "Get"}."Get") -> ("Variable Name Out"=w393:string)  [unwired: 11 in, 6 out]
                n211 = call "GFG_core.vi"("Variable Name in"="experiment type", "Variant in"=T7 "XYT" ("experiment type"), "Action"=enum16{"Init", "Set", "Get"}."Set") -> ()  [unwired: 10 in, 7 out]
                n212 = call-poly "GFGpolyGet.vi"("Variable Name in"="fill.fraction") -> ("output cluster"=w387:T12)  [unwired: 9 in, 1 out]
                n213 = Unbundle By Name(w387) -> ("DigitalRef"=w388:refnum<vi>)
                n214 = call "GFG_core.vi"("Variable Name in"=" no..of.frames.to.acquire", "Variant in"=w393, "Action"=enum16{"Init", "Set", "Get"}."Set") -> ()  [unwired: 10 in, 7 out]
                n215 = call-poly "GFGpolyGet.vi"("Variable Name in"="y.pixels") -> ("output cluster"=w390:T12)  [unwired: 9 in, 1 out]
                n216 = property class="DigNum"(reference=w388, "DisabledEnum"=T4."Enabled" ("Disabled")) -> ()  [unwired: 1 in, 2 out]
                n217 = call "line scan enable disable.vi"("Page Enabled State"=T8."Page Disabled & Grayed") -> ()  [unwired: 11 in]
                n218 = Unbundle By Name(w390) -> ("DigitalRef"=w389:refnum<vi>)
                n219 = property class="DigNum"(reference=w389, "DisabledEnum"=T4."Enabled" ("Disabled")) -> ()  [unwired: 1 in, 2 out]
              }
              frame "Z Stack" {
                n220 = call "GFG_core.vi"("Variable Name in"="advanced settings inner tab", "Variant in"=advanced_settings_inner_tab_CTL."Zstack data" ("advanced settings inner tab"), "Action"=enum16{"Init", "Set", "Get"}."Set") -> ()  [unwired: 10 in, 7 out]
                n221 = call "GFG_core.vi"("Variable Name in"="experiment type", "Variant in"=T7 "XYTZ" ("experiment type"), "Action"=enum16{"Init", "Set", "Get"}."Set") -> ()  [unwired: 10 in, 7 out]
                n222 = call "control tab sliding.vi"("close(T)/open(F)"=FALSE, "String"="advanced settings slider tab") -> ()  [unwired: 10 in]
                n223 = call "GFG refresh all variables.vi"("All Variable Names"=string[] ["frames.per.plane"]) -> ()  [unwired: 11 in]
              }
              frame "2D line scan" {
                n224 = call "GFG_core.vi"("Variable Name in"="experiment type", "Variant in"=T7 "[xy]T" ("experiment type"), "Action"=enum16{"Init", "Set", "Get"}."Set") -> ()  [unwired: 10 in, 7 out]
              }
            }
          }
          frame "MAIN.Image.panels." {
            n225 = Variant To Data(type=MAIN_Image_panel_tab_Control_type_def."Channel 1" ("MAIN Image panels"), Variant=w422) -> (data=w421:T10)  [unwired: 1 in, 1 out]
            n226 = case shown="\"all channels\"" w421 {
              tunnel: w420 -> [w424 w426 w428 w430 w436]
              tunnel: [w424 w426 w428 w430 w436] -> w419
              tunnel: [Histogram_tab."hist Ch 1" ("Histograms tab") Histogram_tab."hist Ch 2" ("Histograms tab") Histogram_tab."hist Ch 3" ("Histograms tab") Histogram_tab."hist Ch 4" ("Histograms tab") Histogram_tab."hist Ch 1" ("Histograms tab")] -> w414
              frame "Channel 1", Default {
              }
              frame "Channel 2" {
              }
              frame "Channel 3" {
              }
              frame "Channel 4" {
              }
              frame "all channels" {
                n227 = call-poly "GFGpolyGet.vi"() -> ("DisplayRefsOut(generic class)"=w435:T13)  [unwired: 10 in, 1 out]
                n228 = call-poly "GFGpolyGet.vi"() -> ("Image Refs Out"=w434:T15)  [unwired: 10 in, 1 out]
                n229 = Cluster To Array(cluster=w435) -> (array=w433:refnum<vi>[])
                n230 = Cluster To Array(cluster=w434) -> (array=w432:T14[])
                n231 = call "set initial zoom.vi"("reset?"=TRUE, "Image Refs In"=w432, "DisplayRefsIn(generic class)"=w433) -> ()  [unwired: 9 in]
              }
            }
            n232 = call-poly "GFGpolyGet.vi"("Variable Name in"="Histograms tab") -> ("output cluster"=w417:T12)  [unwired: 9 in, 1 out]
            n233 = Unbundle By Name(w417) -> ("TabControlRef"=w415:refnum<vi>)
            n234 = property class="TabCtl"(reference=w415, "Value"=w414) -> ()  [unwired: 1 in, 2 out]
          }
          frame "Objective" {
            n235 = Variant To Data(type=u16 0, Variant=w456) -> (data=w438:u16)  [unwired: 1 in, 1 out]
            n236 = Increment(x=w438) -> (x+1=w450:u16)
            n237 = Number To Decimal String(number=w450) -> (decimal integer string=w443:string)  [unwired: 1 in]
            n238 = call "GFG_core.vi"("Variable Name in"="active.objective", "Variant in"=w438, "Action"=enum16{"Init", "Set", "Get"}."Set") -> ()  [unwired: 10 in, 7 out]
            n239 = Concatenate Strings("obj", w443, ".max.field.of.view") -> (w451:string)
            n240 = Concatenate Strings("obj", w443, ".voltage.for.max.field.of.view") -> (w444:string)
            n241 = call-poly "GFGpolyGet.vi"("Variable Name in"=w451) -> ("Numeric"=w448:dbl)  [unwired: 9 in, 1 out]
            n242 = call-poly "GFGpolyGet.vi"("Variable Name in"=w444) -> ("Numeric"=w441:dbl)  [unwired: 9 in, 1 out]
            n243 = call "GFG_core.vi"("Variable Name in"="max.field.of.view", "Variant in"=w448, "Action"=enum16{"Init", "Set", "Get"}."Set") -> ()  [unwired: 10 in, 7 out]
            n244 = call "GFG_core.vi"("Variable Name in"="voltage.for.max.field.of.view", "Variant in"=w441, "Action"=enum16{"Init", "Set", "Get"}."Set") -> ()  [unwired: 10 in, 7 out]
          }
          frame "shutdown" {
          }
        }
      }
    }
  }
